vi "FPGA Target_PCIe_7856R.vi"() -> ()   [LabVIEW 2023]
uses:
  <vilib>/Platform/TimedLoop/XDataNode/timing_clust.ctl
  <vilib>/Platform/TimedLoop/XDataNode/nitl_modes.ctl
  <vilib>/Platform/TimedLoop/XDataNode/wakeup.ctl
  <vilib>/rvi/Emulation/niFpgaSctlEmulationGetInTimedLoop.vi
  <vilib>/rvi/Emulation/niFpgaProcessEmulError.vi
  <vilib>/rvi/eio/common/nirviEmuTemplateMethod_errors.vi
  <vilib>/rvi/Emulation/niFpgaGetClockAttributes.vi
  <vilib>/rvi/Emulation/niFpgaEmulationReportErrorSimple.vi
  <vilib>/eio/utilities/niEioResolveVilibRelativePath.vi
  <vilib>/rvi/interface/RandomDataEmulation/niFpgaRandomDataHandleErrors.vi
  <vilib>/rvi/Emulation/niFpgaCriticalErrorInLSC.vi
  Tick Count.vi
  <vilib>/rvi/Memory/Memory_Emulation/nirvimemoryFastEmulation.vi
  <vilib>/rvi/Memory/Memory_Emulation/nirvimemoryEmulation.vi
  <vilib>/rvi/Emulation/niFpgaEmulationIsFPGAContextNoSignature.vi
  <vilib>/rvi/DataTransferAndStorage/Container/Common/niFpgaContainerGetUniqueNameForEmu.vi
  <vilib>/rvi/errors/nirviReportUnexpectedCaseInternalError (U32).vi
  <vilib>/eio/EIONode/EIONode.xnode
  <vilib>/rvi/DataTransferAndStorage/Container/XNode/niFpgaContainer.xnode
  <vilib>/rvi/interface/RandomDataEmulation/nirviRandomDataFpgaReadWriteTemplate.vi
  <vilib>/Platform/TimedLoop/XDataNode/XDataNode.xnode
  <vilib>/rvi/Arithmetic/AddSubMult/XNode/nirviSatArithmetic.xnode
  <vilib>/Platform/TimedLoop/XDataNode/XDNodeRunTimeDep.lvlib
panel:
  out "Move Z Picomotor Direction":bool
  out "Move Z Picomotor":bool
  out "Tick Count(Ticks)":u32
  in  "HoldTimerScale":u64=18446744073709526080
  in  "Feedback1 on  Hold":bool
  out "Feedback2 Error":i32
  out "Feedback1 Error":i32
  out "Feedback2 Boolean":bool
  out "Feedback1 Boolean":bool
  out "ExtraTime 4":fxp<+,64,64>
  in  "DistanceToBulk 3":i16
  in  "DistanceToBulk 2":i16
  out "HasHeldHoldTimeHappend?":bool
  out "Z_axis_-10Vto10V":bool
  out "TraceRetraceFirstUse":bool
  in  "DistanceToBulk":i16
  out "V START":i16
  out "V END":i16
  out "X START":i16
  out "Y START":i16
  out "Z START":i16
  out "X END":i16
  out "Y END":i16
  out "Z END":i16
  out "V2 START":i16
  out "Count Average":i16
  out "AverageSum":i64
  out "IterateHolder":i16
  out "V2 VEl":i16
  out "V2 END":i16
  out "Update Position Loop Wait Time (ms)":u16=1
  out "LineType":i16
  out "V VEl":i16
  out "Z VEL":i16
  out "Y VEL":i16
  out "X VEL":i16
  out "Element":i16
  in  "V on Fly":i16=-32768
  in  "Change V on Fly":bool
  in  "Feedback_Threshold":i64
  in  "FeedBackType":u8
  out "x < y?":bool
  out "ExtraTime 3":fxp<+,64,64>
  in  "P2AvgMinus":i32
  out "ExtraTime 2":fxp<+,64,64>
  in  "P2AvgWhole":i32
  in  "Xoffset":u32
  in  "P":fxp<+/-,32,1>
  in  "Upper limit Of dZ":i32
  in  "FeedBackType 2":u8
  in  "Feedback_Threshold 2":i32
  in  "GreaterThan 2":bool
  in  "GreaterThan":bool
  in  "V2 on Fly":i16=-32768
  in  "Change V on Fly 2":bool
  out "CurrentMeasuredX":i16
  in  "2^(-n)":i16
  out "SampleNum":i16
  in  "Buffer Loop Wait Time (tICKS)":u32=1
  out "SampleIterator":i16
  out "Internal Stop":bool caption="Stop"
  out "MeasuredCurrent":i16=32767
  out "Applied Voltage":i16=-32768
  in  "External Stop":bool caption="Stop"
  in  "External Pause":bool
  out "Applied Z":i16
  out "Applied Y":i16
  out "Applied X":i16
  in  "Internal Pause":bool
  out "Accum Z":i32
  out "Accum I":i32
  out "Accum dV":i32
  out "Accum I2":i32
  out "OnlyStopLineONCE X":bool
  out "Accum Ext ac":i32
  out "Ext amp":i16=32767
  out "Accum Ext phase":i32
  in  "ExpandVelScaller X":i16=-27
  out "LineNumber":u64
  out "WaitingForWayPoints":bool caption="Stop"
  out "HoldTimer (ticks)":u64
  out "MeasuredCurrent 2":i16=32767
  out "Ext Phase":i16=32767
  in  "ExpandVelScaller Y":i16=-27
  in  "ExpandVelScaller Z":i16=-27
  in  "ExpandVelScaller V":i16=-27
  out "Accum I3":i32
  out "MeasuredCurrent 3":i16=32767
  out "MeasuredCurrent 4":i16=32767
  out "Accum Y":i32
  out "Accum X":i32
  out "OnlyStopLineONCE Y":bool
  out "OnlyStopLineONCE Z":bool
  out "OnlyStopLineONCE V":bool
  in  "EndCurrentLine":bool
  out "StopMoveX":bool
  out "StopMoveY":bool
  out "StopMoveZ":bool
  out "StopMoveV":bool
  out "Jump V":bool
  out "Stop Hold Position":bool
  out "Applied Voltage 2":i16
  out "StopMoveV2":bool
  out "Accum dV2":i32
  out "Jump V2":bool
  in  "ExpandVelScaller V2":i16=-27
  out "OnlyStopLineONCE V2":bool
  out "MoveAverage":i16
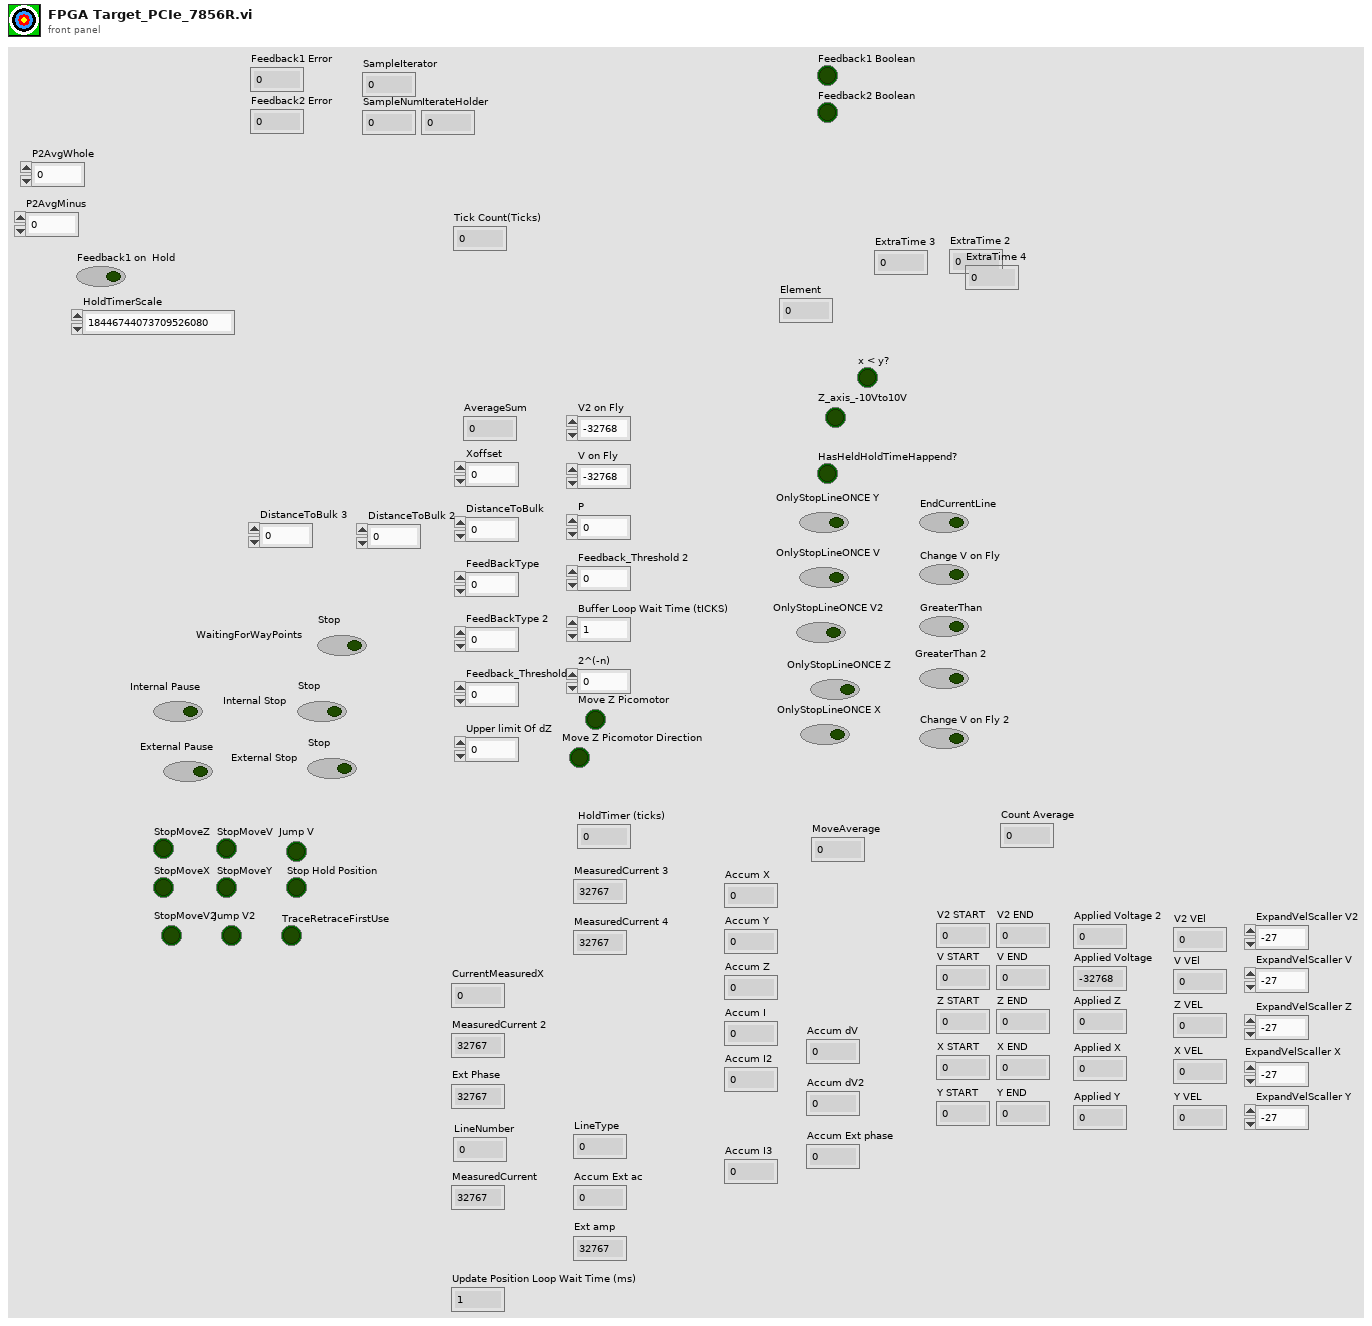
[diagram p1: front panel]
types:
  T1 = typedef "XDNodeRunTimeDep.lvlib/timing_clust.ctl" = cluster{"Expected End [f-1]":u64, "Actual End [f-1]":u64, "Finished Late? [f-1]":bool, "Expected End [i-1]":u64, "Actual End [i-1]":u64, "Finished Late? [i-1]":bool, "Expected Start [i]":u64, "Actual Start [i]":u64, "Expected Start [f]":u64, "Actual Start [f]":u64, "Source Name":string, "Structure Name":string, "Period":i64, "Deadline":i64, "Offset":i64, "Start":i64, "Priority":i32, "Timeout":i32, "Mode":T2, "Wakeup Reason":T3, "Error":errorcluster, "Source Type":string, "Secondary Source Type":string, "Global End Time":u64, "Global Start Time":u64, "Frame Duration":u64, "Iteration Duration":u64, "Assigned CPU":i32, "I/O Scan Engine Mode":u32}
  T2 = typedef "XDNodeRunTimeDep.lvlib/nitl_modes.ctl" = enum32{"No Change", "Process missed periods, maintain original phase", "Discard missed periods, maintain original phase", "Process missed periods, ignore original phase", "Discard missed periods, ignore original phase"}
  T3 = typedef "XDNodeRunTimeDep.lvlib/wakeup.ctl" = enum32{"Normal", "Aborted", "Asynchronous wakeup", "Timing source error", "Timed loop error", "Timeout"}
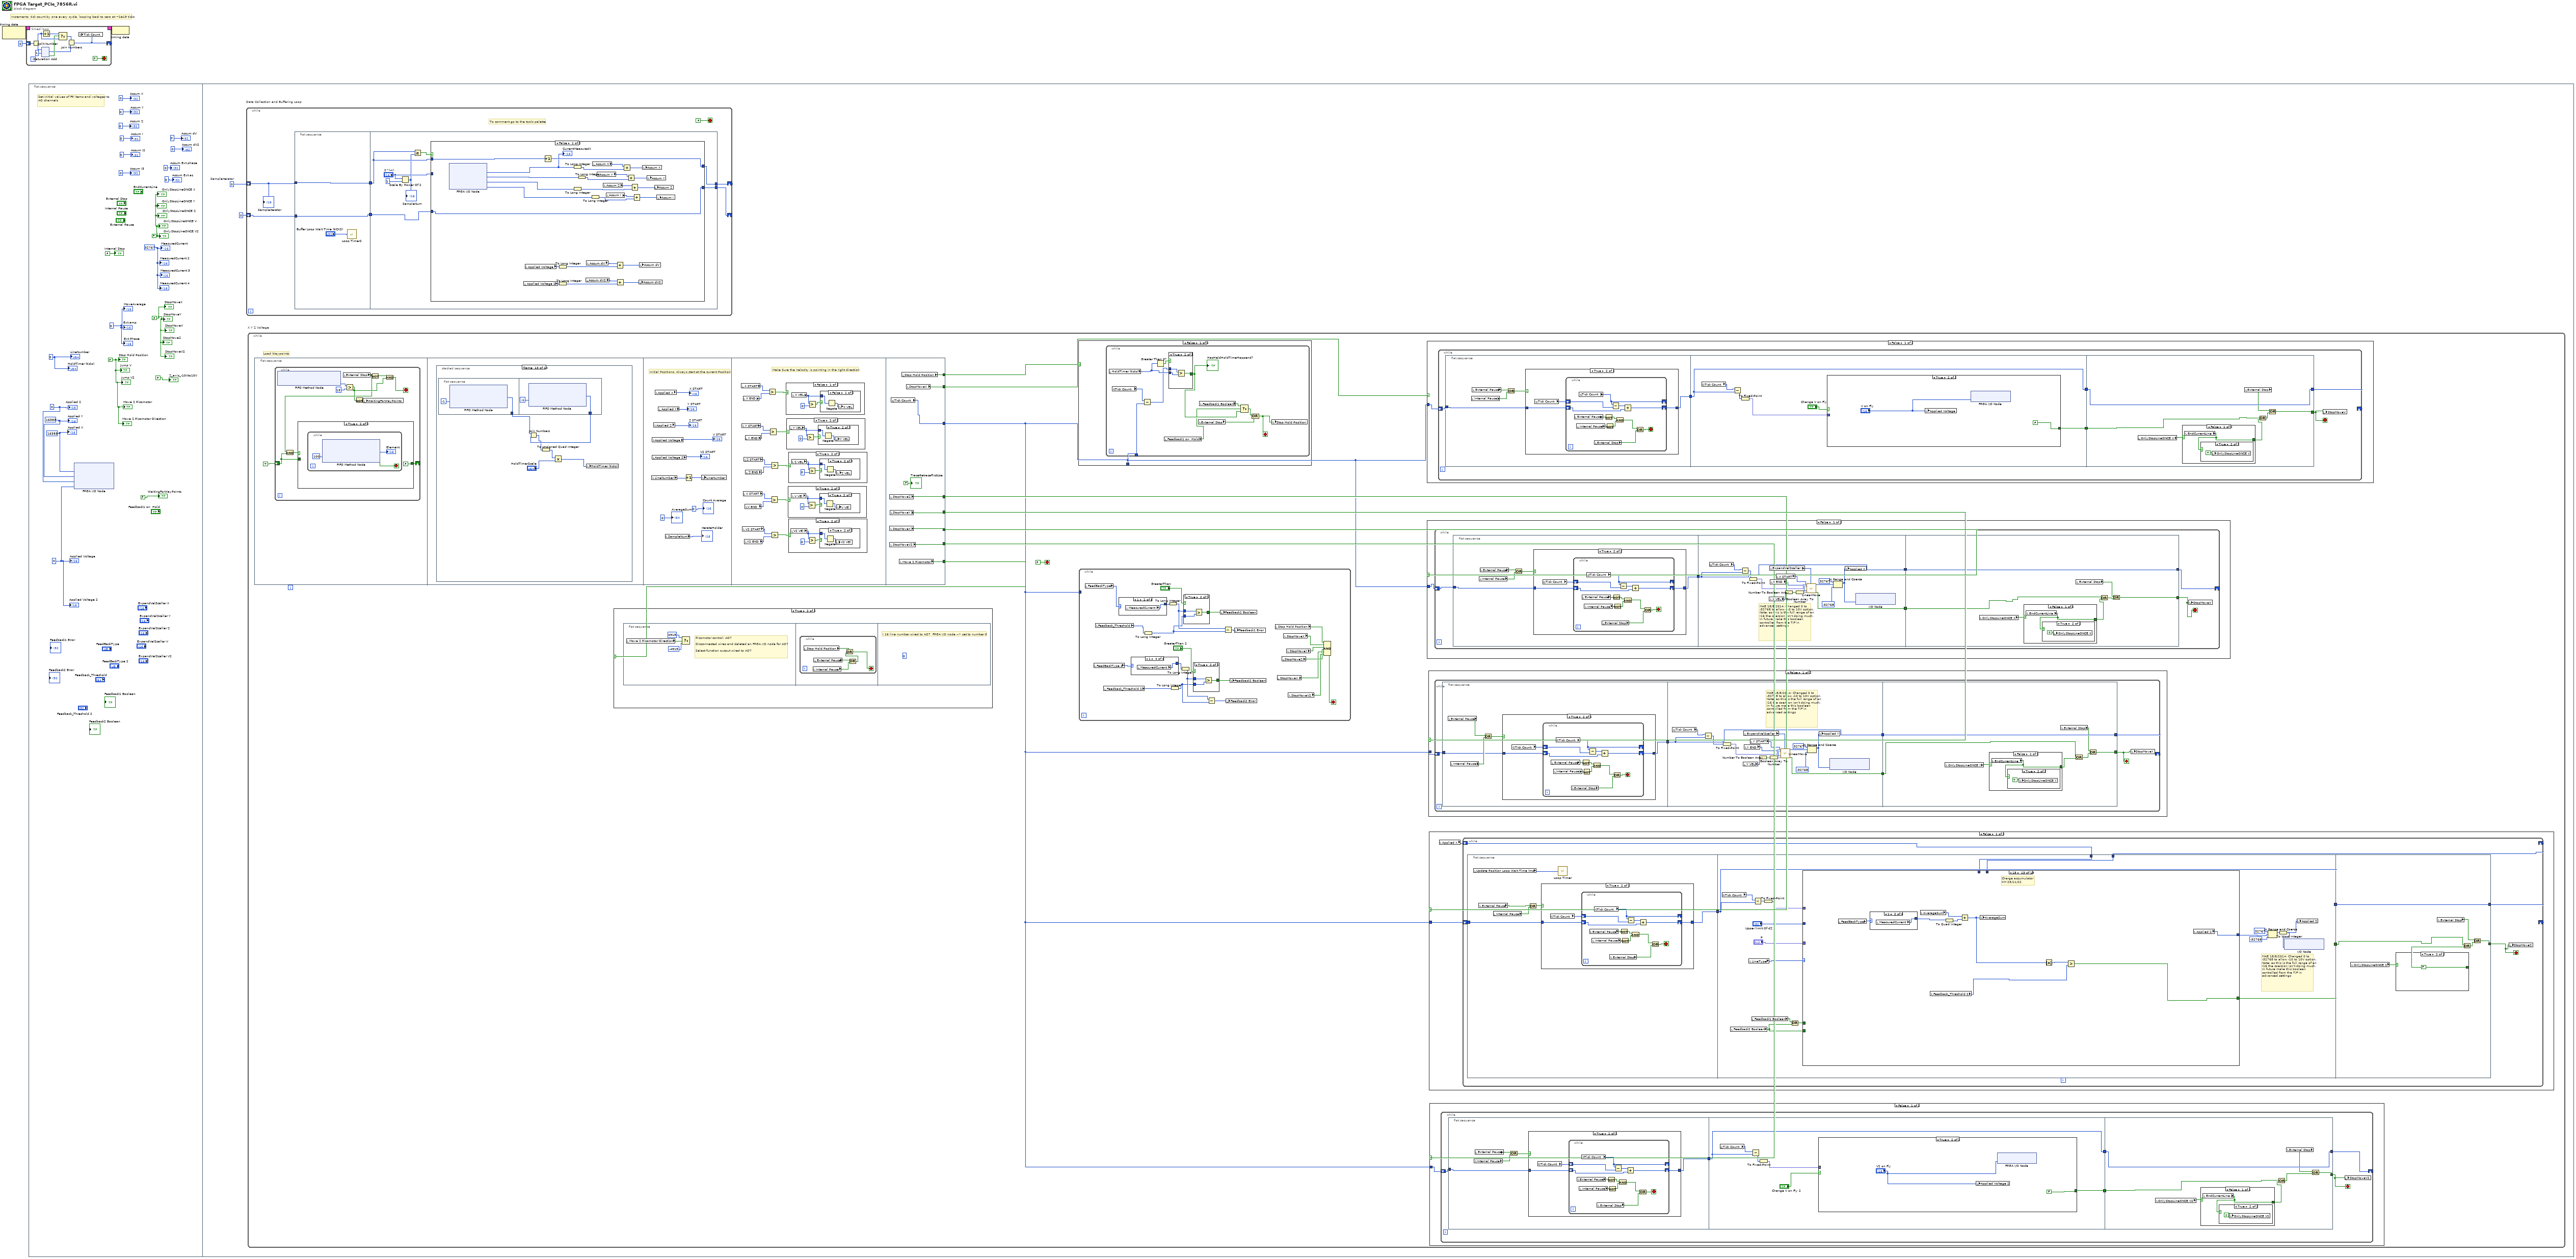
[diagram p0: block diagram]
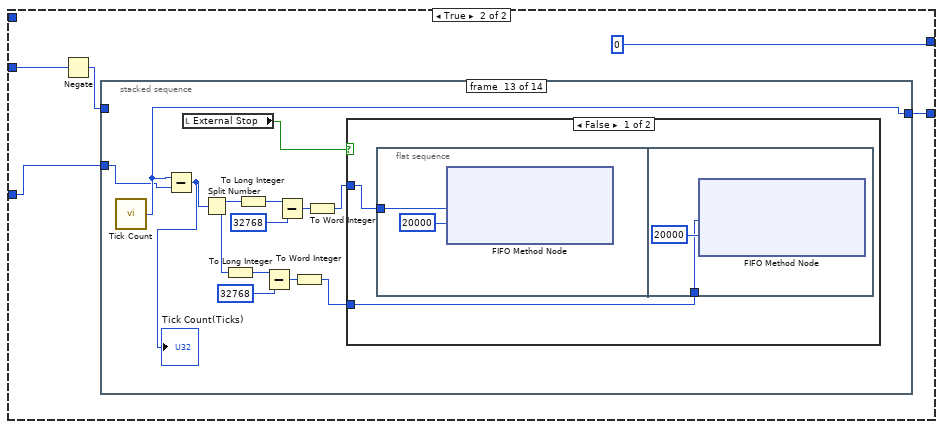
[diagram p2: hidden frame]
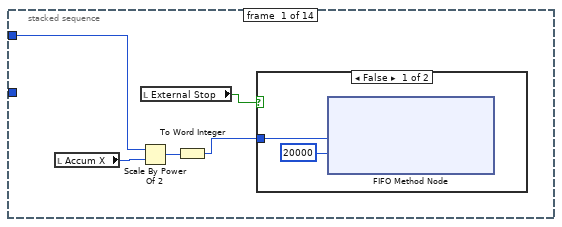
[diagram p3: hidden frame]
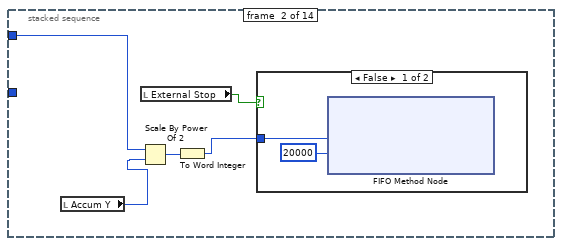
[diagram p5: hidden frame]
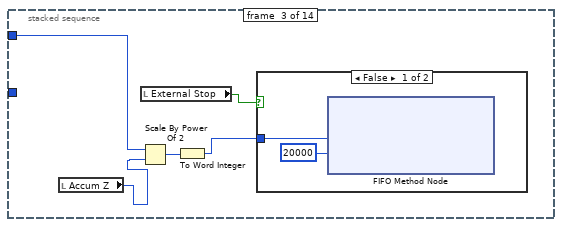
[diagram p7: hidden frame]
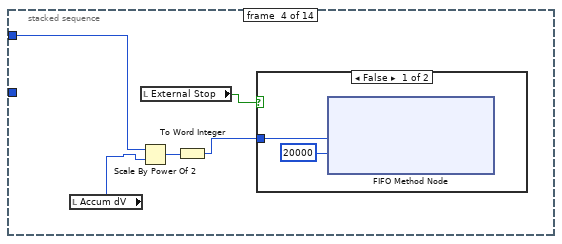
[diagram p9: hidden frame]
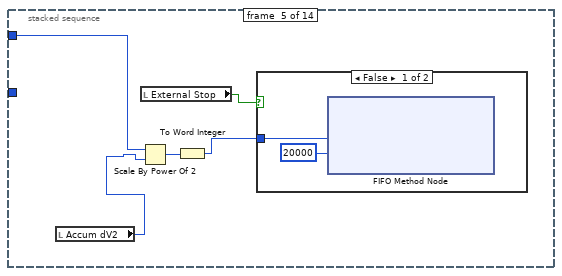
[diagram p11: hidden frame]
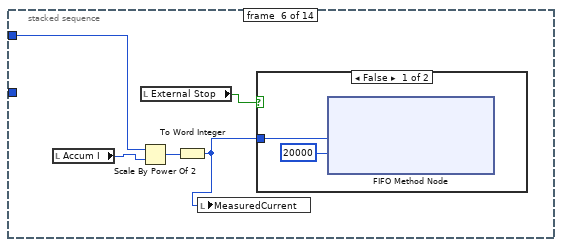
[diagram p13: hidden frame]
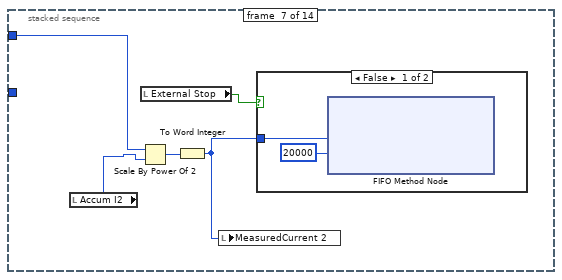
[diagram p15: hidden frame]
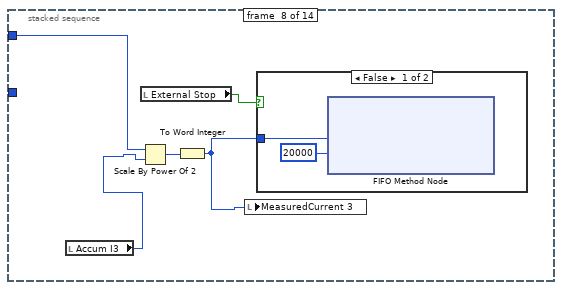
[diagram p17: hidden frame]
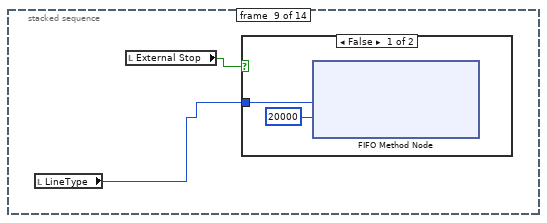
[diagram p19: hidden frame]
diagram:
  # "Increments  tick count by one every cycle, looping back to zero at ~2e19 ticks"
  n1 = node-c288() -> (w3:T1)  [unwired: 1 in]
  n2 = timed-loop {
    timing: w3 -> [_]
    timing-out: [_] -> w2
    shift-right: [w5] -> _
    shift-left: u64 0 -> [w13]
    stop <- FALSE stop-if-true
    n3 = Split Number(x=w13) -> (hi(x)=w10:u32, lo(x)=w12:u32)
    n4 = xnode "Saturation Add"("x"=w12, "y"=u32 1) -> ("x+y"=w6:u32, "overflow"=w7:bool)
    n5 = Increment(x=w10) -> (x+1=w11:u32)
    n6 = Select(t=w11, s=w7, f=w10) -> (s? t:f=w9:u32)
    n7 = Join Numbers(hi=w9, lo=w6) -> ((hi.lo)=w5:u64)
    n8 = global write "Tick Count.vi" "Tick Count"(w5) -> ()
  }
  n9 = flat-sequence {
    frame #0 {
      w33 = FALSE ("OnlyStopLineONCE V2")
      w34 = FALSE ("Internal Stop")
      w29 = FALSE ("Internal Stop")
      w36 = i16 0 ("Applied Volatge")
      w37 = i16 16383 ("Applied Volatge")
      w38 = i16 16383 ("Applied Volatge")
      w32 = u64 0 ("LineNumber")
      w31 = i16 0 ("Ext amp")
      w28 = i16 0 ("Applied Volatge")
      w41 = i16 32767 ("dZ Position")
      # "Set initial values of FP items and voltages to AO channels"
      n10 = xnode "FPGA I/O Node"("Connector0/AO0"=w38, "Connector0/AO1"=w37, "Connector0/AO2"=w36, "Connector0/AO4"=w28) -> ()  [unwired: 4 in, 4 out]
      "Internal Stop" <- FALSE ("Internal Stop")
      "MeasuredCurrent" <- w41
      "Applied Voltage" <- w28
      "Applied Z" <- w36
      "Applied Y" <- w37
      "Applied X" <- w38
      "Accum Z" <- 0 ("Applied Volatge")
      "Accum I" <- 0 ("Applied Volatge")
      "Accum dV" <- 0 ("Applied Volatge")
      "Accum I2" <- 0 ("Applied Volatge")
      "OnlyStopLineONCE X" <- w33
      "Accum Ext ac" <- 0 ("Accum Ext ac")
      "Ext amp" <- w31
      "Accum Ext phase" <- 0 ("Accum Ext phase")
      "LineNumber" <- w32
      "WaitingForWayPoints" <- FALSE ("WaitingForWayPoints")
      "HoldTimer (ticks)" <- w32
      "MeasuredCurrent 2" <- w41
      "Ext Phase" <- w31
      "Accum I3" <- 0 ("Applied Volatge")
      "MeasuredCurrent 3" <- w41
      "MeasuredCurrent 4" <- w41
      "Accum Y" <- 0 ("Applied Volatge")
      "Accum X" <- 0 ("Applied Volatge")
      "OnlyStopLineONCE Y" <- w33
      "OnlyStopLineONCE Z" <- w33
      "OnlyStopLineONCE V" <- w33
      "StopMoveX" <- w34
      "StopMoveY" <- w34
      "StopMoveZ" <- w34
      "StopMoveV" <- w34
      "Jump V" <- w29
      "Stop Hold Position" <- w29
      "Applied Voltage 2" <- w28
      "StopMoveV2" <- w34
      "Accum dV2" <- 0 ("Applied Volatge")
      "Jump V2" <- w29
      "OnlyStopLineONCE V2" <- w33
      "MoveAverage" <- w31
      "Z_axis_-10Vto10V" <- FALSE ("Internal Stop")
      "Move Z Picomotor" <- w29
      "Move Z Picomotor Direction" <- w29
    }
    frame #1 {
      w52 = i16 0  # SampleIterator
      n11 = while "Data Collection and Buffering Loop" {
        shift-right: [w57] -> _
        shift-left: w52 -> [w58]
        shift-right: [w55] -> _
        shift-left: u32 0 ("Tick Count(Ticks)") -> [w53]
        stop <- FALSE stop-if-true
        # "To comment go to the tools palette"
        n12 = flat-sequence {
          tunnel: [w62] -> w59
          tunnel: w58 -> [w62]
          tunnel: w53 -> [w60]
          tunnel: [w60] -> w54
          tunnel: w59 -> [w70]
          tunnel: [w69] -> w57
          tunnel: [w64] -> w55
          tunnel: w54 -> [w63]
          frame #0 {
            n13 = call "Loop Timer2"("Count(Ticks)"="Buffer Loop Wait Time (tICKS)") -> ()  [unwired: 1 out]
          }
          frame #1 {
            n14 = Scale By Power Of 2(n="2^(-n)", x=i16 1) -> (x*2^n=w67:i16)
            "SampleNum" <- w67
            n15 = Greater Or Equal?(x=w70, y=w67) -> (x >= y?=w65:bool)
            n16 = case shown="False" w65 {
              tunnel: w70 -> [w97 _]
              tunnel: [w96 i16 0 ("lo")] -> w69
              tunnel: "2^(-n)" -> [_ w101]
              tunnel: [w72 w99] -> w64
              tunnel: w63 -> [w72 w98]
              frame False {
                n17 = xnode "FPGA I/O Node"() -> ("Connector0/AI0"=w77:i16, "Connector0/AI1"=w84:i16, "Connector0/AI2"=w87:i16, "Connector0/AI4"=w71:i16)  [unwired: 4 in, 4 out]
                "CurrentMeasuredX" <- w77
                n18 = local read "Applied Voltage 2"() -> (w75:i16)
                n19 = local read "Applied Voltage"() -> (w89:i16)
                n20 = Increment(x=w97) -> (x+1=w96:i16)
                n21 = To Long Integer(number=w89) -> (32bit integer=w88:i32)
                n22 = To Long Integer(number=w75) -> (32bit integer=w76:i32)
                n23 = To Long Integer(number=w87) -> (32bit integer=w85:i32)
                n24 = To Long Integer(number=w77) -> (32bit integer=w78:i32)
                n25 = To Long Integer(number=w84) -> (32bit integer=w83:i32)
                n26 = local read "Accum dV2"() -> (w73:i32)
                n27 = local read "Accum dV"() -> (w91:i32)
                n28 = To Long Integer(number=w71) -> (32bit integer=w93:i32)
                n29 = local read "Accum X"() -> (w79:i32)
                n30 = local read "Accum Y"() -> (w82:i32)
                n31 = local read "Accum Z"() -> (w86:i32)
                n32 = local read "Accum I"() -> (w94:i32)
                n33 = Add(x=w91, y=w88) -> (x+y=w90:i32)
                n34 = Add(x=w73, y=w76) -> (x+y=w74:i32)
                n35 = Add(x=w79, y=w78) -> (x+y=w80:i32)
                n36 = Add(x=w82, y=w83) -> (x+y=w81:i32)
                n37 = Add(x=w86, y=w85) -> (x+y=w95:i32)
                n38 = Add(x=w94, y=w93) -> (x+y=w92:i32)
                n39 = local write "Accum dV2"(w74) -> ()
                n40 = local write "Accum dV"(w90) -> ()
                n41 = local write "Accum X"(w80) -> ()
                n42 = local write "Accum Y"(w81) -> ()
                n43 = local write "Accum Z"(w95) -> ()
                n44 = local write "Accum I"(w92) -> ()
              }
              frame True {
                n45 = Negate(x=w101) -> (-x=w100:i16)
                n46 = stacked-sequence {
                  tunnel: w100 -> [w103 w111 w118 w126 w133 w140 w147 w154 _ _ w171 w178 _ _]
                  tunnel: [_ _ _ _ _ _ _ _ _ _ _ _ w184 _] -> w99
                  tunnel: w98 -> [_ _ _ _ _ _ _ _ _ _ _ _ w183 _]
                  frame #0 {
                    n47 = local read "Accum X"() -> (w104:i32)
                    n48 = Scale By Power Of 2(n=w103, x=w104) -> (x*2^n=w105:i32)
                    n49 = local read "External Stop"() -> (w106:bool)
                    n50 = To Word Integer(number=w105) -> (16bit integer=w107:i16)
                    n51 = case shown="False" w106 {
                      tunnel: w107 -> [w108 _]
                      frame False {
                        n52 = xnode ("FIFO Method Node")("Element"=w108, "Timeout"=20000) -> ()  [unwired: 1 in, 2 out]
                      }
                      frame True {
                      }
                    }
                  }
                  frame #1 {
                    n53 = local read "Accum Y"() -> (w110:i32)
                    n54 = Scale By Power Of 2(n=w111, x=w110) -> (x*2^n=w112:i32)
                    n55 = local read "External Stop"() -> (w113:bool)
                    n56 = To Word Integer(number=w112) -> (16bit integer=w114:i16)
                    n57 = case shown="False" w113 {
                      tunnel: w114 -> [w115 _]
                      frame False {
                        n58 = xnode ("FIFO Method Node")("Element"=w115, "Timeout"=20000) -> ()  [unwired: 1 in, 2 out]
                      }
                      frame True {
                      }
                    }
                  }
                  frame #2 {
                    n59 = local read "Accum Z"() -> (w117:i32)
                    n60 = Scale By Power Of 2(n=w118, x=w117) -> (x*2^n=w119:i32)
                    n61 = local read "External Stop"() -> (w120:bool)
                    n62 = To Word Integer(number=w119) -> (16bit integer=w121:i16)
                    n63 = case shown="False" w120 {
                      tunnel: w121 -> [w122 _]
                      frame False {
                        n64 = xnode ("FIFO Method Node")("Element"=w122, "Timeout"=20000) -> ()  [unwired: 1 in, 2 out]
                      }
                      frame True {
                      }
                    }
                  }
                  frame #3 {
                    n65 = local read "Accum dV"() -> (w124:i32)
                    n66 = Scale By Power Of 2(n=w126, x=w124) -> (x*2^n=w127:i32)
                    n67 = local read "External Stop"() -> (w128:bool)
                    n68 = To Word Integer(number=w127) -> (16bit integer=w125:i16)
                    n69 = case shown="False" w128 {
                      tunnel: w125 -> [w129 _]
                      frame False {
                        n70 = xnode ("FIFO Method Node")("Element"=w129, "Timeout"=20000) -> ()  [unwired: 1 in, 2 out]
                      }
                      frame True {
                      }
                    }
                  }
                  frame #4 {
                    n71 = local read "Accum dV2"() -> (w131:i32)
                    n72 = Scale By Power Of 2(n=w133, x=w131) -> (x*2^n=w134:i32)
                    n73 = local read "External Stop"() -> (w135:bool)
                    n74 = To Word Integer(number=w134) -> (16bit integer=w132:i16)
                    n75 = case shown="False" w135 {
                      tunnel: w132 -> [w136 _]
                      frame False {
                        n76 = xnode ("FIFO Method Node")("Element"=w136, "Timeout"=20000) -> ()  [unwired: 1 in, 2 out]
                      }
                      frame True {
                      }
                    }
                  }
                  frame #5 {
                    n77 = local read "Accum I"() -> (w139:i32)
                    n78 = Scale By Power Of 2(n=w140, x=w139) -> (x*2^n=w141:i32)
                    n79 = local read "External Stop"() -> (w142:bool)
                    n80 = To Word Integer(number=w141) -> (16bit integer=w138:i16)
                    n81 = local write "MeasuredCurrent"(w138) -> ()
                    n82 = case shown="False" w142 {
                      tunnel: w138 -> [w143 _]
                      frame False {
                        n83 = xnode ("FIFO Method Node")("Element"=w143, "Timeout"=20000) -> ()  [unwired: 1 in, 2 out]
                      }
                      frame True {
                      }
                    }
                  }
                  frame #6 {
                    n84 = local read "Accum I2"() -> (w146:i32)
                    n85 = Scale By Power Of 2(n=w147, x=w146) -> (x*2^n=w148:i32)
                    n86 = local read "External Stop"() -> (w149:bool)
                    n87 = To Word Integer(number=w148) -> (16bit integer=w145:i16)
                    n88 = local write "MeasuredCurrent 2"(w145) -> ()
                    n89 = case shown="False" w149 {
                      tunnel: w145 -> [w150 _]
                      frame False {
                        n90 = xnode ("FIFO Method Node")("Element"=w150, "Timeout"=20000) -> ()  [unwired: 1 in, 2 out]
                      }
                      frame True {
                      }
                    }
                  }
                  frame #7 {
                    n91 = local read "Accum I3"() -> (w153:i32)
                    n92 = Scale By Power Of 2(n=w154, x=w153) -> (x*2^n=w155:i32)
                    n93 = local read "External Stop"() -> (w156:bool)
                    n94 = To Word Integer(number=w155) -> (16bit integer=w152:i16)
                    n95 = local write "MeasuredCurrent 3"(w152) -> ()
                    n96 = case shown="False" w156 {
                      tunnel: w152 -> [w157 _]
                      frame False {
                        n97 = xnode ("FIFO Method Node")("Element"=w157, "Timeout"=20000) -> ()  [unwired: 1 in, 2 out]
                      }
                      frame True {
                      }
                    }
                  }
                  frame #8 {
                    n98 = local read "LineType"() -> (w159:i16)
                    n99 = local read "External Stop"() -> (w160:bool)
                    n100 = case shown="False" w160 {
                      tunnel: w159 -> [w161 _]
                      frame False {
                        n101 = xnode ("FIFO Method Node")("Element"=w161, "Timeout"=20000) -> ()  [unwired: 1 in, 2 out]
                      }
                      frame True {
                      }
                    }
                  }
                  frame #9 {
                    n102 = local read "LineNumber"() -> (w164:u64)
                    n103 = local read "External Stop"() -> (w165:bool)
                    n104 = To Word Integer(number=w164) -> (16bit integer=w163:i16)
                    n105 = case shown="False" w165 {
                      tunnel: w163 -> [w166 _]
                      frame False {
                        n106 = xnode ("FIFO Method Node")("Element"=w166, "Timeout"=20000) -> ()  [unwired: 1 in, 2 out]
                      }
                      frame True {
                      }
                    }
                  }
                  frame #10 {
                    n107 = local read "Accum Ext ac"() -> (w170:i32)
                    n108 = local read "External Stop"() -> (w172:bool)
                    n109 = Scale By Power Of 2(n=w171, x=w170) -> (x*2^n=w169:i32)
                    n110 = To Word Integer(number=w169) -> (16bit integer=w168:i16)
                    n111 = case shown="False" w172 {
                      tunnel: w168 -> [w173 _]
                      frame False {
                        n112 = xnode ("FIFO Method Node")("Element"=w173, "Timeout"=20000) -> ()  [unwired: 1 in, 2 out]
                      }
                      frame True {
                      }
                    }
                    n113 = local write "Ext amp"(w168) -> ()
                  }
                  frame #11 {
                    n114 = local read "Accum Ext phase"() -> (w176:i32)
                    n115 = local read "External Stop"() -> (w179:bool)
                    n116 = Scale By Power Of 2(n=w178, x=w176) -> (x*2^n=w177:i32)
                    n117 = To Word Integer(number=w177) -> (16bit integer=w175:i16)
                    n118 = local write "Ext Phase"(w175) -> ()
                    n119 = case shown="False" w179 {
                      tunnel: w175 -> [w180 _]
                      frame False {
                        n120 = xnode ("FIFO Method Node")("Element"=w180, "Timeout"=20000) -> ()  [unwired: 1 in, 2 out]
                      }
                      frame True {
                      }
                    }
                  }
                  frame #12 {
                    n121 = call "Tick Count"() -> ("Tick Count(Ticks)"=w184:u32)
                    n122 = Subtract(x=w184, y=w183) -> (x-y=w182:u32)
                    "Tick Count(Ticks)" <- w182
                    n123 = local read "External Stop"() -> (w195:bool)
                    n124 = Split Number(x=w182) -> (hi(x)=w194:u16, lo(x)=w186:u16)
                    n125 = To Long Integer(number=w186) -> (32bit integer=w187:i32)
                    n126 = To Long Integer(number=w194) -> (32bit integer=w193:i32)
                    n127 = Subtract(x=w187, y=32768) -> (x-y=w189:i32)
                    n128 = Subtract(x=w193, y=32768) -> (x-y=w191:i32)
                    n129 = To Word Integer(number=w189) -> (16bit integer=w185:i16)
                    n130 = To Word Integer(number=w191) -> (16bit integer=w190:i16)
                    n131 = case shown="False" w195 {
                      tunnel: w190 -> [w197 _]
                      tunnel: w185 -> [w196 _]
                      frame False {
                        n132 = flat-sequence {
                          tunnel: w197 -> [w198]
                          tunnel: w196 -> [w200]
                          frame #0 {
                            n133 = xnode ("FIFO Method Node")("Element"=w198, "Timeout"=20000) -> ()  [unwired: 1 in, 2 out]
                          }
                          frame #1 {
                            n134 = xnode ("FIFO Method Node")("Element"=w200, "Timeout"=20000) -> ()  [unwired: 1 in, 2 out]
                          }
                        }
                      }
                      frame True {
                      }
                    }
                  }
                  frame #13 {
                    n135 = local write "Accum dV"(0 ("MeasuredCurrent")) -> ()
                    n136 = local write "Accum Z"(0 ("MeasuredCurrent")) -> ()
                    n137 = local write "Accum dV2"(0 ("Accum Ext ac")) -> ()
                    n138 = local write "Accum I2"(0 ("MeasuredCurrent")) -> ()
                    n139 = local write "Accum I"(0 ("MeasuredCurrent")) -> ()
                    n140 = local write "Accum Y"(0 ("Accum Ext ac")) -> ()
                    n141 = local write "Accum X"(0 ("MeasuredCurrent")) -> ()
                    n142 = local write "Accum Ext ac"(0 ("Accum Ext ac")) -> ()
                    n143 = local write "Accum I3"(0 ("Accum Ext ac")) -> ()
                    n144 = local write "Accum Ext phase"(0 ("Accum Ext phase")) -> ()
                  }
                }
              }
            }
          }
        }
        "SampleIterator" <- w58
      }
      n145 = while "X Y Z Voltage" {
        stop <- FALSE stop-if-true
        # "Load Waypoints"
        n146 = flat-sequence {
          tunnel: [w1138] -> w213
          tunnel: [w1137] -> w219
          tunnel: [w1136] -> w218
          tunnel: [w1135] -> w217
          tunnel: [w1134] -> w216
          tunnel: [w1133] -> w215
          tunnel: [w1131] -> w214
          tunnel: [w1130] -> w212
          frame #0 {
            n147 = while {
              shift-right: [w934] -> _
              shift-left: TRUE ("WaitingForWayPoints") -> [w935]
              stop <- w938 stop-if-true
              n148 = xnode ("FIFO Method Node")() -> ("Number of Elements to Read"=w943:u32)  [unwired: 1 in, 1 out]
              n149 = local read "External Stop"() -> (w936:bool)
              n150 = And(x=w936, y=w935) -> (x .and. y?=w937:bool)
              n151 = case shown="True" w937 {
                tunnel: w935 -> [w944 _]
                tunnel: [w944 FALSE ("WaitingForWayPoints")] -> w934
                frame False {
                }
                frame True {
                  n152 = while {
                    stop <- w946 stop-if-true
                    n153 = xnode ("FIFO Method Node")("Timeout"=100) -> ("Element"=→"Element":i16, "Timed Out?"=w946:bool)  [unwired: 1 in, 1 out]
                  }
                }
              }
              n154 = Greater?(x=w943, y=u32 13) -> (0:w939:bool)
              n155 = Not(x=w939) -> (.not. x?=w941:bool)
              n156 = local write "WaitingForWayPoints"(w941) -> ()
              n157 = Not(x=w936) -> (.not. x?=w940:bool)
              n158 = And(x=w940, y=w939) -> (x .and. y?=w938:bool)
            }
          }
          frame #1 {
            n159 = stacked-sequence {
              frame #0 {
                n160 = xnode ("FIFO Method Node")("Timeout"=-1) -> ("Element"=→"LineType":i16)  [unwired: 1 in, 2 out]
              }
              frame #1 {
                n161 = xnode ("FIFO Method Node")("Timeout"=-1) -> ("Element"=→"X VEL":i16)  [unwired: 1 in, 2 out]
              }
              frame #2 {
                n162 = xnode ("FIFO Method Node")("Timeout"=-1) -> ("Element"=→"Y VEL":i16)  [unwired: 1 in, 2 out]
              }
              frame #3 {
                n163 = xnode ("FIFO Method Node")("Timeout"=-1) -> ("Element"=→"Z VEL":i16)  [unwired: 1 in, 2 out]
              }
              frame #4 {
                n164 = xnode ("FIFO Method Node")("Timeout"=-1) -> ("Element"=→"V VEl":i16)  [unwired: 1 in, 2 out]
              }
              frame #5 {
                n165 = xnode ("FIFO Method Node")("Timeout"=-1) -> ("Element"=→"V2 VEl":i16)  [unwired: 1 in, 2 out]
              }
              frame #6 {
                n166 = xnode ("FIFO Method Node")("Timeout"=-1) -> ("Element"=→"X END":i16)  [unwired: 1 in, 2 out]
              }
              frame #7 {
                n167 = xnode ("FIFO Method Node")("Timeout"=-1) -> ("Element"=→"Y END":i16)  [unwired: 1 in, 2 out]
              }
              frame #8 {
                n168 = xnode ("FIFO Method Node")("Timeout"=-1) -> ("Element"=w966:i16)  [unwired: 1 in, 2 out]
                n169 = local read "LineType"() -> (w967:i16)
                n170 = case shown="13" w967 {
                  tunnel: [w969 w974 w986 w998 w1006] -> w965
                  tunnel: w966 -> [w969 _ _ _ _]
                  frame 0..2, Default {
                    # "Normal Move"
                  }
                  frame 3 {
                    # "Bulk At End Of line - Retract"
                    n171 = local read "Z_axis_-10Vto10V"() -> (w973:bool)
                    n172 = local read "Applied Z"() -> (w981:i16)
                    n173 = Select(t=-32768 ("lower limit"), s=w973, f=0 ("lower limit")) -> (s? t:f=w972:i32)
                    n174 = To Long Integer(number=w981) -> (32bit integer=w978:i32)
                    n175 = To Long Integer(number="DistanceToBulk") -> (32bit integer=w979:i32)
                    n176 = Add(x=w978, y=w979) -> (x+y=w977:i32)
                    n177 = In Range and Coerce(upper limit=32767, x=w977, lower limit=w972) -> (coerced(x)=w975:i32)  [unwired: 1 out]
                    n178 = To Word Integer(number=w975) -> (16bit integer=w974:i16)
                  }
                  frame 12 {
                    # "Bulk At End Of line - Retract"
                    n179 = local read "Z_axis_-10Vto10V"() -> (w985:bool)
                    n180 = local read "Applied Z"() -> (w993:i16)
                    n181 = Select(t=-32768 ("lower limit"), s=w985, f=0 ("lower limit")) -> (s? t:f=w984:i32)
                    n182 = To Long Integer(number=w993) -> (32bit integer=w990:i32)
                    n183 = To Long Integer(number="DistanceToBulk 2") -> (32bit integer=w991:i32)
                    n184 = Add(x=w990, y=w991) -> (x+y=w989:i32)
                    n185 = In Range and Coerce(upper limit=32767, x=w989, lower limit=w984) -> (coerced(x)=w987:i32)  [unwired: 1 out]
                    n186 = To Word Integer(number=w987) -> (16bit integer=w986:i16)
                  }
                  frame 13 {
                    # "Bulk At End Of line - Retract"
                    n187 = local read "Z_axis_-10Vto10V"() -> (w997:bool)
                    n188 = local read "Applied Z"() -> (w1005:i16)
                    n189 = Select(t=-32768 ("lower limit"), s=w997, f=0 ("lower limit")) -> (s? t:f=w996:i32)
                    n190 = To Long Integer(number=w1005) -> (32bit integer=w1002:i32)
                    n191 = To Long Integer(number="DistanceToBulk 3") -> (32bit integer=w1003:i32)
                    n192 = Add(x=w1002, y=w1003) -> (x+y=w1001:i32)
                    n193 = In Range and Coerce(upper limit=32767, x=w1001, lower limit=w996) -> (coerced(x)=w999:i32)  [unwired: 1 out]
                    n194 = To Word Integer(number=w999) -> (16bit integer=w998:i16)
                  }
                  frame 4..7 {
                    # "Start at current hieght"
                    n195 = local read "Applied Z"() -> (w1006:i16)
                  }
                }
                "Z END" <- w965
              }
              frame #9 {
                n196 = xnode ("FIFO Method Node")("Timeout"=-1) -> ("Element"=→"V END":i16)  [unwired: 1 in, 2 out]
              }
              frame #10 {
                n197 = xnode ("FIFO Method Node")("Timeout"=-1) -> ("Element"=→"V2 END":i16)  [unwired: 1 in, 2 out]
              }
              frame #11 {
                n198 = xnode ("FIFO Method Node")("Timeout"=-1) -> ("Element"=w1012:i16)  [unwired: 1 in, 2 out]
                n199 = To Unsigned Word Integer(number=w1012) -> (unsigned 16bit integer=→"Update Position Loop Wait Time (ms)":u16)
              }
              frame #12 {
                n200 = flat-sequence {
                  tunnel: [w1020] -> w1016
                  tunnel: [w1022] -> w1015
                  frame #0 {
                    n201 = xnode ("FIFO Method Node")("Timeout"=-1) -> ("Element"=w1020:i16)  [unwired: 1 in, 2 out]
                  }
                  frame #1 {
                    n202 = xnode ("FIFO Method Node")("Timeout"=-1) -> ("Element"=w1022:i16)  [unwired: 1 in, 2 out]
                  }
                }
                n203 = Join Numbers(hi=w1016, lo=w1015) -> ((hi.lo)=w1014:u32)
                n204 = To Unsigned Quad Integer(1:w1014) -> (0:w1019:u64)
                n205 = Multiply(x=w1019, y="HoldTimerScale") -> (x*y=w1017:u64)
                n206 = local write "HoldTimer (ticks)"(w1017) -> ()
              }
              frame #13 {
                n207 = xnode ("FIFO Method Node")("Timeout"=-1) -> ("Element"=w1033:i16)  [unwired: 1 in, 2 out]
                n208 = Number To Boolean Array(number=w1033) -> (Boolean array=w1024:bool[])
                n209 = Index Array(array=w1024, index=0) -> (element=w1038:bool)
                n210 = Index Array(array=w1024, index=1) -> (element=w1039:bool)
                n211 = Index Array(array=w1024, index=2) -> (element=w1043:bool)
                n212 = Index Array(array=w1024, index=4) -> (element=w1048:bool)
                n213 = Index Array(array=w1024, index=5) -> (element=w1032:bool)
                n214 = Index Array(array=w1024, index=3) -> (element=w1040:bool)
                n215 = Index Array(array=w1024, index=10) -> (element=w1026:bool)
                n216 = Index Array(array=w1024, index=9) -> (element=w1027:bool)
                n217 = Index Array(array=w1024, index=6) -> (element=w1050:bool)
                n218 = Not(x=w1040) -> (.not. x?=w1047:bool)
                n219 = Not(x=w1038) -> (.not. x?=w1044:bool)
                n220 = Not(x=w1032) -> (.not. x?=w1031:bool)
                n221 = Index Array(array=w1024, index=7) -> (element=w1053:bool)
                n222 = Index Array(array=w1024, index=8) -> (element=w1029:bool)
                n223 = Not(x=w1043) -> (.not. x?=w1046:bool)
                n224 = Not(x=w1039) -> (.not. x?=w1045:bool)
                n225 = local write "StopMoveX"(w1044) -> ()
                n226 = local write "Stop Hold Position"(w1031) -> ()
                n227 = Not(x=w1050) -> (.not. x?=w1051:bool)
                n228 = local write "Move Z Picomotor Direction"(w1026) -> ()
                n229 = local write "StopMoveY"(w1045) -> ()
                n230 = local write "StopMoveZ"(w1046) -> ()
                n231 = local write "StopMoveV2"(w1051) -> ()
                n232 = local write "StopMoveV"(w1047) -> ()
                n233 = local write "Move Z Picomotor"(w1027) -> ()
                n234 = local write "Jump V"(w1048) -> ()
                n235 = local write "Feedback1 on  Hold"(w1029) -> ()
                n236 = local write "Jump V2"(w1053) -> ()
              }
            }
          }
          frame #2 {
            # "Initial Positions, Always start at the current Position"
            n237 = local read "LineNumber"() -> (w1060:u64)
            n238 = local read "Applied Voltage"() -> (→"V START":i16)
            n239 = local read "Applied Voltage 2"() -> (→"V2 START":i16)
            n240 = local read "Applied Z"() -> (→"Z START":i16)
            n241 = local read "Applied X"() -> (→"X START":i16)
            n242 = local read "Applied Y"() -> (→"Y START":i16)
            n243 = local read "SampleNum"() -> (→"IterateHolder":i16)
            n244 = Increment(x=w1060) -> (x+1=w1059:u64)
            n245 = local write "LineNumber"(w1059) -> ()
            "Count Average" <- i16 0
            "AverageSum" <- i64 0 ("LineNumber")
          }
          frame #3 {
            # "Make Sure the Velocity is pointing in the right direction"
            n246 = local read "X START"() -> (w1079:i16)
            n247 = local read "Y START"() -> (w1074:i16)
            n248 = local read "V2 START"() -> (w1067:i16)
            n249 = local read "X END"() -> (w1078:i16)
            n250 = local read "V START"() -> (w1068:i16)
            n251 = local read "Z START"() -> (w1073:i16)
            n252 = local read "V2 END"() -> (w1066:i16)
            n253 = local read "V END"() -> (w1069:i16)
            n254 = local read "Y END"() -> (w1075:i16)
            n255 = local read "Z END"() -> (w1072:i16)
            n256 = Greater?(x=w1079, y=w1078) -> (0:w1077:bool)
            n257 = Greater?(x=w1074, y=w1075) -> (0:w1076:bool)
            n258 = Greater?(x=w1068, y=w1069) -> (0:w1070:bool)
            n259 = Greater?(x=w1073, y=w1072) -> (0:w1071:bool)
            n260 = Greater?(x=w1067, y=w1066) -> (0:w1065:bool)
            n261 = case shown="False" w1077 {
              frame False {
                n262 = local read "X VEL"() -> (w1120:i16)
                n263 = Greater?(x=w1120, y=i16 0) -> (0:w1121:bool)
                n264 = case shown="False" w1121 {
                  tunnel: w1120 -> [w1124 _]
                  frame False {
                    n265 = Negate(x=w1124) -> (-x=w1123:i16)
                    n266 = local write "X VEL"(w1123) -> ()
                  }
                  frame True {
                  }
                }
              }
              frame True {
                n267 = local read "X VEL"() -> (w1125:i16)
                n268 = Greater?(x=w1125, y=i16 0) -> (0:w1126:bool)
                n269 = case shown="True" w1126 {
                  tunnel: w1125 -> [_ w1129]
                  frame False {
                  }
                  frame True {
                    n270 = Negate(x=w1129) -> (-x=w1128:i16)
                    n271 = local write "X VEL"(w1128) -> ()
                  }
                }
              }
            }
            n272 = case shown="True" w1076 {
              frame False {
                n273 = local read "Y VEL"() -> (w1110:i16)
                n274 = Greater?(x=w1110, y=i16 0) -> (0:w1111:bool)
                n275 = case shown="False" w1111 {
                  tunnel: w1110 -> [w1114 _]
                  frame False {
                    n276 = Negate(x=w1114) -> (-x=w1113:i16)
                    n277 = local write "Y VEL"(w1113) -> ()
                  }
                  frame True {
                  }
                }
              }
              frame True {
                n278 = local read "Y VEL"() -> (w1115:i16)
                n279 = Greater?(x=w1115, y=i16 0) -> (0:w1116:bool)
                n280 = case shown="True" w1116 {
                  tunnel: w1115 -> [_ w1119]
                  frame False {
                  }
                  frame True {
                    n281 = Negate(x=w1119) -> (-x=w1118:i16)
                    n282 = local write "Y VEL"(w1118) -> ()
                  }
                }
              }
            }
            n283 = case shown="True" w1070 {
              frame False {
                n284 = local read "V VEl"() -> (w1090:i16)
                n285 = Greater?(x=w1090, y=i16 0) -> (0:w1091:bool)
                n286 = case shown="False" w1091 {
                  tunnel: w1090 -> [w1094 _]
                  frame False {
                    n287 = Negate(x=w1094) -> (-x=w1093:i16)
                    n288 = local write "V VEl"(w1093) -> ()
                  }
                  frame True {
                  }
                }
              }
              frame True {
                n289 = local read "V VEl"() -> (w1095:i16)
                n290 = Greater?(x=w1095, y=i16 0) -> (0:w1096:bool)
                n291 = case shown="True" w1096 {
                  tunnel: w1095 -> [_ w1099]
                  frame False {
                  }
                  frame True {
                    n292 = Negate(x=w1099) -> (-x=w1098:i16)
                    n293 = local write "V VEl"(w1098) -> ()
                  }
                }
              }
            }
            n294 = case shown="True" w1071 {
              frame False {
                n295 = local read "Z VEL"() -> (w1100:i16)
                n296 = Greater?(x=w1100, y=i16 0) -> (0:w1101:bool)
                n297 = case shown="False" w1101 {
                  tunnel: w1100 -> [w1104 _]
                  frame False {
                    n298 = Negate(x=w1104) -> (-x=w1103:i16)
                    n299 = local write "Z VEL"(w1103) -> ()
                  }
                  frame True {
                  }
                }
              }
              frame True {
                n300 = local read "Z VEL"() -> (w1105:i16)
                n301 = Greater?(x=w1105, y=i16 0) -> (0:w1106:bool)
                n302 = case shown="True" w1106 {
                  tunnel: w1105 -> [_ w1109]
                  frame False {
                  }
                  frame True {
                    n303 = Negate(x=w1109) -> (-x=w1108:i16)
                    n304 = local write "Z VEL"(w1108) -> ()
                  }
                }
              }
            }
            n305 = case shown="True" w1065 {
              frame False {
                n306 = local read "V2 VEl"() -> (w1080:i16)
                n307 = Greater?(x=w1080, y=i16 0) -> (0:w1081:bool)
                n308 = case shown="False" w1081 {
                  tunnel: w1080 -> [w1084 _]
                  frame False {
                    n309 = Negate(x=w1084) -> (-x=w1083:i16)
                    n310 = local write "V2 VEl"(w1083) -> ()
                  }
                  frame True {
                  }
                }
              }
              frame True {
                n311 = local read "V2 VEl"() -> (w1085:i16)
                n312 = Greater?(x=w1085, y=i16 0) -> (0:w1086:bool)
                n313 = case shown="True" w1086 {
                  tunnel: w1085 -> [_ w1089]
                  frame False {
                  }
                  frame True {
                    n314 = Negate(x=w1089) -> (-x=w1088:i16)
                    n315 = local write "V2 VEl"(w1088) -> ()
                  }
                }
              }
            }
          }
          frame #4 {
            n316 = local read "StopMoveZ"() -> (w1134:bool)
            n317 = local read "StopMoveX"() -> (w1136:bool)
            n318 = local read "StopMoveV2"() -> (w1133:bool)
            n319 = local read "StopMoveY"() -> (w1135:bool)
            n320 = global read "Tick Count.vi" "Tick Count"() -> (w1138:u64)
            n321 = local read "Move Z Picomotor"() -> (w1130:bool)
            n322 = local read "Stop Hold Position"() -> (w1131:bool)
            n323 = local read "StopMoveV"() -> (w1137:bool)
            "TraceRetraceFirstUse" <- FALSE ("Boolean")
          }
        }
        n324 = case shown="True" w212 {
          frame False {
          }
          frame True {
            n325 = flat-sequence {
              frame #0 {
                # "Picomotor control: AO7\n\nDisconnected wires and deleted an FPGA I/O node for AO7\n\nSelect function output wired to AO7"
                n326 = local read "Move Z Picomotor Direction"() -> (w221:bool)
                n327 = Select(t=i16 4915 ("LineNumber"), s=w221, f=i16 -4915 ("LineNumber")) -> ()  [unwired: 1 out]
              }
              frame #1 {
                n328 = while {
                  stop <- w224 stop-if-true
                  n329 = local read "Stop Hold Position"() -> (w228:bool)
                  n330 = local read "Internal Pause"() -> (w227:bool)
                  n331 = local read "External Pause"() -> (w226:bool)
                  n332 = Or(x=w226, y=w227) -> (x .or. y?=w225:bool)
                  n333 = Or(x=w228, y=w225) -> (x .or. y?=w224:bool)
                }
              }
              frame #2 {
                (unwired) i16 0 ("LineNumber")
                # "I 16 line number wired to AO7  FPGA I/O node --> set to number 0"
              }
            }
          }
        }
        n334 = case shown="False" w214 {
          tunnel: w213 -> [w276 _]
          frame False {
            n335 = while {
              tunnel: w276 -> [w284]
              stop <- w280 stop-if-true
              n336 = local read "HoldTimer (ticks)"() -> (w286:u64)
              n337 = global read "Tick Count.vi" "Tick Count"() -> (w285:u64)
              n338 = Subtract(x=w285, y=w284) -> (x-y=w283:u64)
              n339 = Greater Than 0?(x=w286) -> (x > 0?=w287:bool)
              n340 = local read "Feedback1 on  Hold"() -> (w277:bool)
              n341 = case shown="True" w287 {
                tunnel: [FALSE w291] -> w278
                tunnel: w286 -> [_ w290]
                tunnel: w283 -> [_ w289]
                frame False {
                }
                frame True {
                  n342 = Greater?(x=w289, y=w290) -> (0:w291:bool)
                }
              }
              "HasHeldHoldTimeHappend?" <- w278
              n343 = local read "External Stop"() -> (w281:bool)
              n344 = local read "Feedback1 Boolean"() -> (w282:bool)
              n345 = Select(t=w282, s=w277, f=w278) -> (s? t:f=w279:bool)
              n346 = Compound Arithmetic op=OR(w279, w281) -> (w280:bool)
              n347 = local write "Stop Hold Position"(w280) -> ()
            }
          }
          frame True {
          }
        }
        n348 = while {
          tunnel: w213 -> [_]
          stop <- w238 stop-if-true
          n349 = local read "FeedBackType"() -> (w250:u8)
          n350 = local read "FeedBackType 2"() -> (w248:u8)
          n351 = local read "Feedback_Threshold"() -> (w232:i64)
          n352 = local read "Feedback_Threshold 2"() -> (w230:i32)
          n353 = case shown="1" w250 {
            tunnel: [w270 w271 w272 w273 w274 w275] -> w251
            frame 0, Default {
              n354 = local read "Ext amp"() -> (w270:i16)
            }
            frame 1 {
              n355 = local read "MeasuredCurrent"() -> (w271:i16)
            }
            frame 2 {
              n356 = local read "MeasuredCurrent 2"() -> (w272:i16)
            }
            frame 3 {
              n357 = local read "Ext Phase"() -> (w273:i16)
            }
            frame 4 {
              n358 = local read "MeasuredCurrent"() -> (w274:i16)
            }
            frame 5 {
              n359 = local read "MeasuredCurrent 2"() -> (w275:i16)
            }
          }
          n360 = case shown="1" w248 {
            tunnel: [w258 w259 w260 w261 w262 w263] -> w246
            frame 0, Default {
              n361 = local read "Ext amp"() -> (w258:i16)
            }
            frame 4 {
              n362 = local read "MeasuredCurrent 3"() -> (w259:i16)
            }
            frame 5 {
              n363 = local read "MeasuredCurrent 4"() -> (w260:i16)
            }
            frame 1 {
              n364 = local read "MeasuredCurrent"() -> (w261:i16)
            }
            frame 2 {
              n365 = local read "MeasuredCurrent 2"() -> (w262:i16)
            }
            frame 3 {
              n366 = local read "Ext Phase"() -> (w263:i16)
            }
          }
          n367 = To Long Integer(number=w232) -> (32bit integer=w231:i32)
          n368 = To Long Integer(number=w251) -> (32bit integer=w236:i32)
          n369 = To Long Integer(number=w230) -> (32bit integer=w229:i32)
          n370 = To Long Integer(number=w246) -> (32bit integer=w234:i32)
          n371 = case shown="True" "GreaterThan" {
            tunnel: w236 -> [w266 w269]
            tunnel: w231 -> [w265 w267]
            tunnel: [w264 w268] -> w245
            frame False {
              n372 = Less?(x=w266, y=w265) -> (x < y?=w264:bool)
            }
            frame True {
              n373 = Greater?(x=w269, y=w267) -> (0:w268:bool)
            }
          }
          n374 = case shown="True" "GreaterThan 2" {
            tunnel: w234 -> [w254 w257]
            tunnel: w229 -> [w253 w255]
            tunnel: [w252 w256] -> w244
            frame False {
              n375 = Less?(x=w254, y=w253) -> (x < y?=w252:bool)
            }
            frame True {
              n376 = Greater?(x=w257, y=w255) -> (0:w256:bool)
            }
          }
          n377 = Subtract(x=w234, y=w229) -> (x-y=w233:i32)
          n378 = local write "Feedback1 Boolean"(w245) -> ()
          n379 = Subtract(x=w236, y=w231) -> (x-y=w235:i32)
          n380 = local write "Feedback2 Error"(w233) -> ()
          n381 = local write "Feedback2 Boolean"(w244) -> ()
          n382 = local write "Feedback1 Error"(w235) -> ()
          n383 = local read "Stop Hold Position"() -> (w237:bool)
          n384 = local read "StopMoveV"() -> (w240:bool)
          n385 = local read "StopMoveZ"() -> (w241:bool)
          n386 = local read "StopMoveX"() -> (w243:bool)
          n387 = local read "StopMoveY"() -> (w242:bool)
          n388 = local read "StopMoveV2"() -> (w239:bool)
          n389 = Compound Arithmetic op=AND(w237, w243, w242, w241, w240, w239) -> (w238:bool)
        }
        n390 = case shown="False" w219 {
          tunnel: w213 -> [w871 _]
          frame False {
            n391 = while {
              shift-right: [w873] -> _
              shift-left: w871 -> [w876]
              stop <- w872 stop-if-true
              n392 = flat-sequence {
                tunnel: w876 -> [w878]
                tunnel: [w879] -> w877
                tunnel: w877 -> [w904]
                tunnel: [w904] -> w875
                tunnel: [w900] -> w874
                tunnel: [w929] -> w873
                tunnel: w875 -> [w929]
                tunnel: w874 -> [w923]
                tunnel: [w924] -> w872
                frame #0 {
                  n393 = local read "Internal Pause"() -> (w881:bool)
                  n394 = local read "External Pause"() -> (w882:bool)
                  n395 = Or(x=w882, y=w881) -> (x .or. y?=w880:bool)
                  n396 = case shown="True" w880 {
                    tunnel: w878 -> [w883 w886]
                    tunnel: [w883 w884] -> w879
                    frame False {
                    }
                    frame True {
                      n397 = global read "Tick Count.vi" "Tick Count"() -> (w885:u64)
                      n398 = while {
                        shift-right: [w898] -> w884
                        shift-left: w886 -> [w890]
                        shift-right: [w893] -> _
                        shift-left: w885 -> [w892]
                        stop <- w887 stop-if-true
                        n399 = local read "External Pause"() -> (w897:bool)
                        n400 = local read "Internal Pause"() -> (w895:bool)
                        n401 = global read "Tick Count.vi" "Tick Count"() -> (w893:u64)
                        n402 = local read "External Stop"() -> (w889:bool)
                        n403 = Not(x=w897) -> (.not. x?=w896:bool)
                        n404 = Not(x=w895) -> (.not. x?=w894:bool)
                        n405 = Subtract(x=w893, y=w892) -> (x-y=w891:u64)
                        n406 = And(x=w896, y=w894) -> (x .and. y?=w888:bool)
                        n407 = Add(x=w891, y=w890) -> (x+y=w898:u64)
                        n408 = Or(x=w888, y=w889) -> (x .or. y?=w887:bool)
                      }
                    }
                  }
                }
                frame #1 {
                  n409 = global read "Tick Count.vi" "Tick Count"() -> (w903:u64)
                  n410 = Subtract(x=w903, y=w904) -> (x-y=w901:u64)
                  n411 = To Fixed-Point(number=w901) -> (fixed-point=w902:fxp<+,64,64>)  [unwired: 1 in]
                  n412 = case shown="True" "Change V on Fly" {
                    tunnel: w902 -> [w909 _]
                    tunnel: [w908 FALSE ("Finished Move")] -> w900
                    frame False {
                      n413 = local read "Jump V"() -> (w907:bool)
                      n414 = local read "V END"() -> (w906:i16)
                      n415 = case shown="True" w907 {
                        tunnel: w906 -> [w918 w919]
                        tunnel: [w917 w919] -> w905
                        tunnel: w909 -> [w916 _]
                        tunnel: [w915 TRUE ("Finished Move")] -> w908
                        frame False {
                          n416 = local read "ExpandVelScaller V"() -> (w910:i16)
                          n417 = local read "V VEl"() -> (w913:i16)
                          n418 = local read "V START"() -> (w914:i16)
                          n419 = Number To Boolean Array(number=w913) -> (Boolean array=w912:bool[])
                          n420 = Boolean Array To Number(Boolean array=w912) -> (number=w911:fxp<+/-,16,16>)
                          n421 = call "LinearMove.vi"("Time"=w916, "Start"=w914, "End"=w918, "Velocity"=w911, "ExpandVelScaller"=w910) -> ("OutPosition"=w917:i16, "Finished Move"=w915:bool)  [unwired: 13 in]
                        }
                        frame True {
                        }
                      }
                      n422 = local write "Applied Voltage"(w905) -> ()
                      n423 = xnode "FPGA I/O Node"("Connector0/AO3"=w905) -> ()  [unwired: 1 in, 1 out]
                    }
                    frame True {
                      n424 = local write "Applied Voltage"("V on Fly") -> ()
                      n425 = xnode "FPGA I/O Node"("Connector0/AO3"="V on Fly") -> ()  [unwired: 1 in, 1 out]
                    }
                  }
                }
                frame #2 {
                  n426 = local read "OnlyStopLineONCE V"() -> (w925:bool)
                  n427 = case shown="False" w925 {
                    tunnel: [w930 FALSE ("EndCurrentLine")] -> w926
                    frame False {
                      n428 = local read "EndCurrentLine"() -> (w930:bool)
                      n429 = case shown="True" w930 {
                        frame False {
                        }
                        frame True {
                          n430 = local write "OnlyStopLineONCE V"(TRUE ("EndCurrentLine")) -> ()
                        }
                      }
                    }
                    frame True {
                    }
                  }
                  n431 = local read "External Stop"() -> (w927:bool)
                  n432 = Or(x=w923, y=w926) -> (x .or. y?=w928:bool)
                  n433 = Or(x=w927, y=w928) -> (x .or. y?=w924:bool)
                }
              }
              n434 = local write "StopMoveV"(w872) -> ()
            }
          }
          frame True {
          }
        }
        n435 = case shown="False" w218 {
          tunnel: w213 -> [w818 _]
          frame False {
            n436 = while {
              shift-right: [w820] -> _
              shift-left: w818 -> [w823]
              stop <- w819 stop-if-true
              n437 = flat-sequence {
                tunnel: w823 -> [w825]
                tunnel: [w826] -> w824
                tunnel: w824 -> [w860]
                tunnel: [w860] -> w822
                tunnel: [w857] -> w821
                tunnel: [w867] -> w820
                tunnel: w822 -> [w867]
                tunnel: w821 -> [w861]
                tunnel: [w862] -> w819
                frame #0 {
                  n438 = local read "Internal Pause"() -> (w828:bool)
                  n439 = local read "External Pause"() -> (w829:bool)
                  n440 = Or(x=w829, y=w828) -> (x .or. y?=w827:bool)
                  n441 = case shown="True" w827 {
                    tunnel: w825 -> [w830 w833]
                    tunnel: [w830 w831] -> w826
                    frame False {
                    }
                    frame True {
                      n442 = global read "Tick Count.vi" "Tick Count"() -> (w832:u64)
                      n443 = while {
                        shift-right: [w845] -> w831
                        shift-left: w833 -> [w837]
                        shift-right: [w840] -> _
                        shift-left: w832 -> [w839]
                        stop <- w834 stop-if-true
                        n444 = local read "External Pause"() -> (w844:bool)
                        n445 = local read "Internal Pause"() -> (w842:bool)
                        n446 = global read "Tick Count.vi" "Tick Count"() -> (w840:u64)
                        n447 = local read "External Stop"() -> (w836:bool)
                        n448 = Not(x=w844) -> (.not. x?=w843:bool)
                        n449 = Not(x=w842) -> (.not. x?=w841:bool)
                        n450 = Subtract(x=w840, y=w839) -> (x-y=w838:u64)
                        n451 = And(x=w843, y=w841) -> (x .and. y?=w835:bool)
                        n452 = Add(x=w838, y=w837) -> (x+y=w845:u64)
                        n453 = Or(x=w835, y=w836) -> (x .or. y?=w834:bool)
                      }
                    }
                  }
                }
                frame #1 {
                  # "MAE 18/8/2014: Changed 0 to -32768 to allow -10 to 10V option. Note: as this is the full range of an I16 the coercion isn't doing much. In future make this boolean controlled from the T/F in advanced settings"
                  n454 = global read "Tick Count.vi" "Tick Count"() -> (w859:u64)
                  n455 = Subtract(x=w859, y=w860) -> (x-y=w846:u64)
                  n456 = To Fixed-Point(number=w846) -> (fixed-point=w858:fxp<+,64,64>)  [unwired: 1 in]
                  n457 = local read "X VEL"() -> (w850:i16)
                  n458 = local read "ExpandVelScaller X"() -> (w847:i16)
                  n459 = local read "X END"() -> (w848:i16)
                  n460 = local read "X START"() -> (w849:i16)
                  n461 = Number To Boolean Array(number=w850) -> (Boolean array=w856:bool[])
                  n462 = Boolean Array To Number(Boolean array=w856) -> (number=w855:fxp<+/-,16,16>)
                  n463 = call "LinearMove.vi"("Time"=w858, "Start"=w849, "End"=w848, "Velocity"=w855, "ExpandVelScaller"=w847) -> ("OutPosition"=w851:i16, "Finished Move"=w857:bool)  [unwired: 13 in]
                  n464 = In Range and Coerce(upper limit=i16 32767, x=w851, lower limit=i16 -32768) -> (coerced(x)=w852:i16)  [unwired: 1 out]
                  n465 = local write "Applied X"(w852) -> ()
                  n466 = xnode "I/O Node"("Connector0/AO0"=w852) -> ()  [unwired: 1 in, 1 out]
                }
                frame #2 {
                  n467 = local read "OnlyStopLineONCE X"() -> (w864:bool)
                  n468 = case shown="False" w864 {
                    tunnel: [w868 FALSE ("EndCurrentLine")] -> w863
                    frame False {
                      n469 = local read "EndCurrentLine"() -> (w868:bool)
                      n470 = case shown="True" w868 {
                        frame False {
                        }
                        frame True {
                          n471 = local write "OnlyStopLineONCE X"(TRUE ("EndCurrentLine")) -> ()
                        }
                      }
                    }
                    frame True {
                    }
                  }
                  n472 = local read "External Stop"() -> (w866:bool)
                  n473 = Or(x=w861, y=w863) -> (x .or. y?=w865:bool)
                  n474 = Or(x=w866, y=w865) -> (x .or. y?=w862:bool)
                }
              }
              n475 = local write "StopMoveX"(w819) -> ()
            }
          }
          frame True {
          }
        }
        n476 = case shown="False" w217 {
          tunnel: w213 -> [w765 _]
          frame False {
            n477 = while {
              shift-right: [w767] -> _
              shift-left: w765 -> [w770]
              stop <- w766 stop-if-true
              n478 = flat-sequence {
                tunnel: w770 -> [w772]
                tunnel: [w773] -> w771
                tunnel: w771 -> [w807]
                tunnel: [w807] -> w769
                tunnel: [w804] -> w768
                tunnel: [w814] -> w767
                tunnel: w769 -> [w814]
                tunnel: w768 -> [w808]
                tunnel: [w809] -> w766
                frame #0 {
                  n479 = local read "External Pause"() -> (w776:bool)
                  n480 = local read "Internal Pause"() -> (w775:bool)
                  n481 = Or(x=w776, y=w775) -> (x .or. y?=w774:bool)
                  n482 = case shown="True" w774 {
                    tunnel: w772 -> [w777 w780]
                    tunnel: [w777 w778] -> w773
                    frame False {
                    }
                    frame True {
                      n483 = global read "Tick Count.vi" "Tick Count"() -> (w779:u64)
                      n484 = while {
                        shift-right: [w792] -> w778
                        shift-left: w780 -> [w784]
                        shift-right: [w787] -> _
                        shift-left: w779 -> [w786]
                        stop <- w781 stop-if-true
                        n485 = local read "External Pause"() -> (w791:bool)
                        n486 = local read "Internal Pause"() -> (w789:bool)
                        n487 = global read "Tick Count.vi" "Tick Count"() -> (w787:u64)
                        n488 = local read "External Stop"() -> (w783:bool)
                        n489 = Not(x=w791) -> (.not. x?=w790:bool)
                        n490 = Not(x=w789) -> (.not. x?=w788:bool)
                        n491 = Subtract(x=w787, y=w786) -> (x-y=w785:u64)
                        n492 = And(x=w790, y=w788) -> (x .and. y?=w782:bool)
                        n493 = Add(x=w785, y=w784) -> (x+y=w792:u64)
                        n494 = Or(x=w782, y=w783) -> (x .or. y?=w781:bool)
                      }
                    }
                  }
                }
                frame #1 {
                  # "MAE 18/8/2014: Changed 0 to -32768 to allow -10 to 10V option. Note: as this is the full range of an I16 the coercion isn't doing much. In future make this boolean controlled from the T/F in advanced settings"
                  n495 = global read "Tick Count.vi" "Tick Count"() -> (w806:u64)
                  n496 = Subtract(x=w806, y=w807) -> (x-y=w793:u64)
                  n497 = To Fixed-Point(number=w793) -> (fixed-point=w805:fxp<+,64,64>)  [unwired: 1 in]
                  n498 = local read "Y VEL"() -> (w797:i16)
                  n499 = local read "ExpandVelScaller Y"() -> (w794:i16)
                  n500 = local read "Y END"() -> (w795:i16)
                  n501 = local read "Y START"() -> (w796:i16)
                  n502 = Number To Boolean Array(number=w797) -> (Boolean array=w803:bool[])
                  n503 = Boolean Array To Number(Boolean array=w803) -> (number=w802:fxp<+/-,16,16>)
                  n504 = call "LinearMove.vi"("Time"=w805, "Start"=w796, "End"=w795, "Velocity"=w802, "ExpandVelScaller"=w794) -> ("OutPosition"=w798:i16, "Finished Move"=w804:bool)  [unwired: 13 in]
                  n505 = In Range and Coerce(upper limit=i16 32767, x=w798, lower limit=i16 -32768) -> (coerced(x)=w799:i16)  [unwired: 1 out]
                  n506 = local write "Applied Y"(w799) -> ()
                  n507 = xnode "I/O Node"("Connector0/AO1"=w799) -> ()  [unwired: 1 in, 1 out]
                }
                frame #2 {
                  n508 = local read "OnlyStopLineONCE Y"() -> (w810:bool)
                  n509 = case shown="False" w810 {
                    tunnel: [w815 FALSE ("EndCurrentLine")] -> w811
                    frame False {
                      n510 = local read "EndCurrentLine"() -> (w815:bool)
                      n511 = case shown="True" w815 {
                        frame False {
                        }
                        frame True {
                          n512 = local write "OnlyStopLineONCE Y"(TRUE ("EndCurrentLine")) -> ()
                        }
                      }
                    }
                    frame True {
                    }
                  }
                  n513 = local read "External Stop"() -> (w813:bool)
                  n514 = Or(x=w808, y=w811) -> (x .or. y?=w812:bool)
                  n515 = Or(x=w813, y=w812) -> (x .or. y?=w809:bool)
                }
              }
              n516 = local write "StopMoveY"(w766) -> ()
            }
          }
          frame True {
          }
        }
        n517 = case shown="False" w216 {
          tunnel: w213 -> [w355 _]
          frame False {
            n518 = local read "Applied X"() -> (w354:i16)
            n519 = while {
              shift-right: [w359] -> _
              shift-left: w355 -> [w362]
              shift-right: [w356] -> _
              shift-left: w354 -> [w357]
              stop <- w358 stop-if-true
              n520 = flat-sequence {
                tunnel: w362 -> [w365]
                tunnel: [w366] -> w363
                tunnel: w363 -> [w403]
                tunnel: [w403] -> w361
                tunnel: [w398] -> w360
                tunnel: w357 -> [w392]
                tunnel: [w391] -> w356
                tunnel: [w761] -> w359
                tunnel: w361 -> [w761]
                tunnel: w360 -> [w755]
                tunnel: [w756] -> w358
                frame #0 {
                  n521 = local read "Update Position Loop Wait Time (ms)"() -> (w364:u16)
                  n522 = local read "External Pause"() -> (w369:bool)
                  n523 = local read "Internal Pause"() -> (w368:bool)
                  n524 = Or(x=w369, y=w368) -> (x .or. y?=w367:bool)
                  n525 = case shown="True" w367 {
                    tunnel: w365 -> [w370 w373]
                    tunnel: [w370 w371] -> w366
                    frame False {
                    }
                    frame True {
                      n526 = global read "Tick Count.vi" "Tick Count"() -> (w372:u64)
                      n527 = while {
                        shift-right: [w385] -> w371
                        shift-left: w373 -> [w377]
                        shift-right: [w380] -> _
                        shift-left: w372 -> [w379]
                        stop <- w374 stop-if-true
                        n528 = local read "External Pause"() -> (w384:bool)
                        n529 = local read "Internal Pause"() -> (w382:bool)
                        n530 = global read "Tick Count.vi" "Tick Count"() -> (w380:u64)
                        n531 = local read "External Stop"() -> (w376:bool)
                        n532 = Not(x=w384) -> (.not. x?=w383:bool)
                        n533 = Not(x=w382) -> (.not. x?=w381:bool)
                        n534 = Subtract(x=w380, y=w379) -> (x-y=w378:u64)
                        n535 = And(x=w383, y=w381) -> (x .and. y?=w375:bool)
                        n536 = Add(x=w378, y=w377) -> (x+y=w385:u64)
                        n537 = Or(x=w375, y=w376) -> (x .or. y?=w374:bool)
                      }
                    }
                  }
                  n538 = call "Loop Timer"("Count(mSec)"=w364) -> ()  [unwired: 1 out]
                }
                frame #1 {
                  # "MAE 18/8/2014: Changed 0 to -32768 to allow -10 to 10V option. Note: as this is the full range of an I16 the coercion isn't doing much. In future make this boolean controlled from the T/F in advanced settings"
                  n539 = global read "Tick Count.vi" "Tick Count"() -> (w402:u64)
                  n540 = local read "Feedback2 Boolean"() -> (w386:bool)
                  n541 = local read "LineType"() -> (w389:i16)
                  n542 = local read "Feedback1 Boolean"() -> (w387:bool)
                  n543 = Subtract(x=w402, y=w403) -> (x-y=w394:u64)
                  n544 = To Fixed-Point(number=w394) -> (fixed-point=w390:fxp<+,64,64>)  [unwired: 1 in]
                  n545 = Or(x=w387, y=w386) -> (x .or. y?=w388:bool)
                  n546 = case shown="15" w389 {
                    tunnel: "P" -> [_ _ _ w439 w451 w467 w488 _ w523 _ _ _ _]
                    tunnel: [w406 w416 w423 w434 w447 w462 w478 w511 w518 w540 w605 w678 w741] -> w398
                    tunnel: [w405 w415 w425 w437 w449 w465 w477 w514 w521 w542 w607 w680 w746] -> w397
                    tunnel: "Upper limit Of dZ" -> [_ _ _ w433 w448 w464 w487 _ w517 _ _ _ _]
                    tunnel: w392 -> [_ _ _ _ _ _ w485 _ _ _ _ _ _]
                    tunnel: [_ _ _ _ _ _ w484 _ _ _ _ _ _] -> w391
                    tunnel: w390 -> [w404 w414 w424 _ _ _ _ _ _ w541 w606 w679 _]
                    tunnel: w388 -> [_ w413 w423 _ _ _ _ _ _ _ _ _ _]
                    tunnel: w386 -> [_ _ _ _ _ _ _ _ w516 _ _ _ _]
                    frame 0, Default {
                      # "Normal Move"
                      n547 = local read "Z VEL"() -> (w409:i16)
                      n548 = local read "ExpandVelScaller Z"() -> (w412:i16)
                      n549 = local read "Z END"() -> (w411:i16)
                      n550 = local read "Z START"() -> (w410:i16)
                      n551 = Number To Boolean Array(number=w409) -> (Boolean array=w407:bool[])
                      n552 = Boolean Array To Number(Boolean array=w407) -> (number=w408:fxp<+/-,16,16>)
                      n553 = call "LinearMove.vi"("Time"=w404, "Start"=w410, "End"=w411, "Velocity"=w408, "ExpandVelScaller"=w412) -> ("OutPosition"=w405:i16, "Finished Move"=w406:bool)  [unwired: 13 in]
                    }
                    frame 1 {
                      # "Pause on Set Point"
                      n554 = local write "Internal Pause"(w413) -> ()
                      n555 = local read "Z VEL"() -> (w419:i16)
                      n556 = local read "ExpandVelScaller Z"() -> (w422:i16)
                      n557 = local read "Z END"() -> (w421:i16)
                      n558 = local read "Z START"() -> (w420:i16)
                      n559 = Number To Boolean Array(number=w419) -> (Boolean array=w417:bool[])
                      n560 = Boolean Array To Number(Boolean array=w417) -> (number=w418:fxp<+/-,16,16>)
                      n561 = call "LinearMove.vi"("Time"=w414, "Start"=w420, "End"=w421, "Velocity"=w418, "ExpandVelScaller"=w422) -> ("OutPosition"=w415:i16, "Finished Move"=w416:bool)  [unwired: 13 in]
                    }
                    frame 2 {
                      # "STOP Current Move on SetPoint"
                      n562 = local read "Z VEL"() -> (w428:i16)
                      n563 = local read "ExpandVelScaller Z"() -> (w431:i16)
                      n564 = local read "Z END"() -> (w430:i16)
                      n565 = local read "Z START"() -> (w429:i16)
                      n566 = Number To Boolean Array(number=w428) -> (Boolean array=w426:bool[])
                      n567 = Boolean Array To Number(Boolean array=w426) -> (number=w427:fxp<+/-,16,16>)
                      n568 = call "LinearMove.vi"("Time"=w424, "Start"=w429, "End"=w430, "Velocity"=w427, "ExpandVelScaller"=w431) -> ("OutPosition"=w425:i16)  [unwired: 13 in, 1 out]
                    }
                    frame 4 {
                      # "For scanning-Propotional Controller for constant distance scanning"
                      n569 = local read "Feedback1 Error"() -> (w432:i32)
                      n570 = Multiply(x=w439, y=w432) -> (x*y=w444:fxp<+/-,64,33>)
                      n571 = To Word Integer(number=w444) -> (16bit integer=w443:i16)
                      n572 = To Long Integer(number=w443) -> (32bit integer=w445:i32)
                      n573 = local read "StopMoveY"() -> (w435:bool)
                      n574 = local read "StopMoveX"() -> (w436:bool)
                      n575 = local read "Applied Z"() -> (w438:i16)
                      n576 = Negate(x=w433) -> (-x=w440:i32)
                      n577 = And(x=w436, y=w435) -> (x .and. y?=w434:bool)
                      n578 = In Range and Coerce(upper limit=w433, x=w445, lower limit=w440) -> (coerced(x)=w441:i32)  [unwired: 1 out]
                      n579 = To Long Integer(number=w438) -> (32bit integer=w442:i32)
                      n580 = Add(x=w442, y=w441) -> (x+y=w437:i32)
                    }
                    frame 11 {
                      # "Dependent on hold time-Propotional Controller for constant distance scanning"
                      n581 = local read "Feedback1 Error"() -> (w446:i32)
                      n582 = Multiply(x=w451, y=w446) -> (x*y=w456:fxp<+/-,64,33>)
                      n583 = To Word Integer(number=w456) -> (16bit integer=w455:i16)
                      n584 = To Long Integer(number=w455) -> (32bit integer=w457:i32)
                      n585 = local read "HasHeldHoldTimeHappend?"() -> (w447:bool)
                      n586 = local read "Applied Z"() -> (w450:i16)
                      n587 = Negate(x=w448) -> (-x=w452:i32)
                      n588 = In Range and Coerce(upper limit=w448, x=w457, lower limit=w452) -> (coerced(x)=w453:i32)  [unwired: 1 out]
                      n589 = To Long Integer(number=w450) -> (32bit integer=w454:i32)
                      n590 = Add(x=w454, y=w453) -> (x+y=w449:i32)
                    }
                    frame 10 {
                      # "deciding the limit of the Z movement (up or down) regardless of the x value"
                      # "convert the difference in siganls to distance in um"
                      # "External signal-Feedback_Threshold"
                      # "Dependent on holdtime-Propotional Controller for constant distance scanning ONLY for POSITIVE"
                      n591 = local read "Feedback1 Error"() -> (w458:i32)
                      n592 = Multiply(x=w467, y=w458) -> (x*y=w471:fxp<+/-,64,33>)
                      n593 = To Word Integer(number=w471) -> (16bit integer=w470:i16)
                      n594 = To Long Integer(number=w470) -> (32bit integer=w472:i32)
                      n595 = Negate(x=w464) -> (-x=w468:i32)
                      n596 = In Range and Coerce(upper limit=w464, x=w472, lower limit=w468) -> (coerced(x)=w460:i32)  [unwired: 1 out]
                      n597 = Less?(x=w460, y=0) -> (x < y?=w461:bool)
                      n598 = local read "HasHeldHoldTimeHappend?"() -> (w462:bool)
                      n599 = case shown="True" w461 {
                        tunnel: w460 -> [_ w474]
                        tunnel: [0 w474] -> w463
                        frame False {
                        }
                        frame True {
                        }
                      }
                      n600 = local read "Applied Z"() -> (w466:i16)
                      n601 = To Long Integer(number=w466) -> (32bit integer=w469:i32)
                      n602 = Add(x=w469, y=w463) -> (x+y=w465:i32)
                    }
                    frame 5 {
                      # "Proportional controller for constant distance scanning - with storing the positions in a buffer"
                      n603 = local read "Feedback1 Error"() -> (w475:i32)
                      n604 = local read "TraceRetraceFirstUse"() -> (w476:bool)
                      n605 = local read "Applied X"() -> (w484:i16)
                      n606 = local read "Applied Z"() -> (w486:i16)
                      n607 = Multiply(x=w488, y=w475) -> (x*y=w490:fxp<+/-,64,33>)
                      n608 = To Word Integer(number=w490) -> (16bit integer=w491:i16)
                      n609 = Subtract(x=w484, y=w485) -> (x-y=w483:i16)
                      n610 = To Long Integer(number=w491) -> (32bit integer=w489:i32)
                      n611 = case shown="False" w476 {
                        tunnel: w483 -> [w503 w506]
                        tunnel: [w502 w506] -> w482
                        tunnel: [w501 w505] -> w481
                        tunnel: w485 -> [w501 w504]
                        frame False {
                          n612 = Increment(x=w503) -> (x+1=w502:i16)
                        }
                        frame True {
                          n613 = Increment(x=w504) -> (x+1=w505:i16)
                        }
                      }
                      n614 = Negate(x=w487) -> (-x=w494:i32)
                      n615 = In Range and Coerce(upper limit=w487, x=w489, lower limit=w494) -> (coerced(x)=w493:i32)  [unwired: 1 out]
                      n616 = To Long Integer(number=w486) -> (32bit integer=w492:i32)
                      n617 = Add(x=w492, y=w493) -> (x+y=w477:i32)
                      n618 = for {
                        N: w482 -> [_]
                        shift-right: [w496] -> _
                        shift-left: w481 -> [w497]
                        tunnel: w477 -> [w500]
                        n619 = To Unsigned Long Integer(number=w497) -> (unsigned 32bit integer=w498:u32)
                        n620 = To Word Integer(number=w500) -> (16bit integer=w499:i16)
                        n621 = local write "TraceRetraceFirstUse"(TRUE ("TraceRetraceFirst?")) -> ()
                        n622 = xnode ("Memory Write")("Address"=w498, "Data"=w499) -> ()  [unwired: 1 in, 1 out]
                        n623 = Increment(x=w497) -> (x+1=w496:i16)
                      }
                      n624 = local read "StopMoveY"() -> (w479:bool)
                      n625 = local read "StopMoveX"() -> (w480:bool)
                      n626 = And(x=w480, y=w479) -> (x .and. y?=w478:bool)
                    }
                    frame 6 {
                      # "retrace the Z positions stored in the buffer, see feedbaack type 5"
                      n627 = local read "Applied X"() -> (w507:i16)
                      n628 = To Unsigned Long Integer(number=w507) -> (unsigned 32bit integer=w510:u32)
                      n629 = Add(x="Xoffset", y=w510) -> (x+y=w508:u32)
                      n630 = xnode ("Memory Read")("Address"=w508) -> ("Data"=w514:i16)  [unwired: 1 in, 1 out]
                      n631 = local read "StopMoveY"() -> (w512:bool)
                      n632 = local read "StopMoveX"() -> (w513:bool)
                      n633 = And(x=w513, y=w512) -> (x .and. y?=w511:bool)
                    }
                    frame 7 {
                      # "Proportianal controller for constant distance scan, with ability to pause based on a secondary signal"
                      n634 = local write "Internal Pause"(w516) -> ()
                      n635 = local read "Feedback1 Error"() -> (w515:i32)
                      n636 = Multiply(x=w523, y=w515) -> (x*y=w528:fxp<+/-,64,33>)
                      n637 = To Word Integer(number=w528) -> (16bit integer=w527:i16)
                      n638 = To Long Integer(number=w527) -> (32bit integer=w529:i32)
                      n639 = local read "StopMoveY"() -> (w519:bool)
                      n640 = local read "StopMoveX"() -> (w520:bool)
                      n641 = local read "Applied Z"() -> (w522:i16)
                      n642 = Negate(x=w517) -> (-x=w524:i32)
                      n643 = And(x=w520, y=w519) -> (x .and. y?=w518:bool)
                      n644 = In Range and Coerce(upper limit=w517, x=w529, lower limit=w524) -> (coerced(x)=w525:i32)  [unwired: 1 out]
                      n645 = To Long Integer(number=w522) -> (32bit integer=w526:i32)
                      n646 = Add(x=w526, y=w525) -> (x+y=w521:i32)
                    }
                    frame 8 {
                      # "Sum of most recent 1024"
                      n647 = local read "FeedBackType"() -> (w532:u8)
                      n648 = local read "Count Average"() -> (w533:i16)
                      n649 = case shown="1" w532 {
                        tunnel: [w545 w546 w547 w548 w549 w550] -> w531
                        frame 0, Default {
                          n650 = local read "Ext amp"() -> (w545:i16)
                        }
                        frame 1 {
                          n651 = local read "MeasuredCurrent"() -> (w546:i16)
                        }
                        frame 2 {
                          n652 = local read "MeasuredCurrent 2"() -> (w547:i16)
                        }
                        frame 3 {
                          n653 = local read "Ext Phase"() -> (w548:i16)
                        }
                        frame 4 {
                          n654 = local read "MeasuredCurrent"() -> (w549:i16)
                        }
                        frame 5 {
                          n655 = local read "MeasuredCurrent 2"() -> (w550:i16)
                        }
                      }
                      n656 = Equal?(x=w533, y="P2AvgWhole") -> (x = y?=w543:bool)
                      n657 = local read "ExtraTime 2"() -> (w536:fxp<+,64,64>)
                      n658 = To Long Integer(number=w531) -> (32bit integer=w530:i32)
                      n659 = local read "AverageSum"() -> (w539:i64)
                      n660 = case shown="True" w543 {
                        tunnel: w530 -> [w559 w580]
                        tunnel: w539 -> [w560 w587]
                        tunnel: [w561 w587] -> w544
                        tunnel: w533 -> [w558 w574]
                        tunnel: [w557 w574] -> w538
                        tunnel: [w556 w588] -> w542
                        tunnel: w541 -> [w554 w582]
                        tunnel: [FALSE w576] -> w540
                        tunnel: [w554 w584] -> w537
                        tunnel: w536 -> [_ w584]
                        tunnel: [w551 w572] -> w535
                        frame False {
                          n661 = local read "SampleIterator"() -> (w551:i16)
                          n662 = local read "IterateHolder"() -> (w553:i16)
                          n663 = Less?(x=w551, y=w553) -> (x < y?=w552:bool)
                          n664 = case shown="True" w552 {
                            tunnel: [w562 w569] -> w561
                            tunnel: w560 -> [w562 w568]
                            tunnel: w559 -> [_ w564]
                            tunnel: w558 -> [w563 w566]
                            tunnel: [w563 w567] -> w557
                            frame False {
                            }
                            frame True {
                              # "Count up to 1024 (start at 0) data points then start moving"
                              n665 = To Quad Integer(1:w564) -> (0:w565:i64)
                              n666 = Increment(x=w566) -> (x+1=w567:i16)
                              n667 = Add(x=w568, y=w565) -> (x+y=w569:i64)
                            }
                          }
                          n668 = local read "Applied Z"() -> (w556:i16)
                        }
                        frame True {
                          # "STOP Current Move on SetPoint"
                          n669 = local read "AverageSum"() -> (w586:i64)
                          n670 = local read "Feedback_Threshold"() -> (w571:i64)
                          n671 = Subtract(x=w582, y=w584) -> (x-y=w585:fxp<+/-,64,65>)
                          n672 = Scale By Power Of 2(n="P2AvgMinus", x=w586) -> (x*2^n=w575:i64)
                          n673 = To Fixed-Point(fixed-point type=w582, number=w585) -> (fixed-point=w583:fxp<+,64,64>)
                          n674 = To Long Integer(number=w571) -> (32bit integer=w570:i32)
                          n675 = local read "Z VEL"() -> (w591:i16)
                          n676 = Subtract(x=w575, y=w570) -> (x-y=w581:i64)
                          n677 = local read "ExpandVelScaller Z"() -> (w594:i16)
                          n678 = local read "Z END"() -> (w593:i16)
                          n679 = local read "Z START"() -> (w592:i16)
                          n680 = Number To Boolean Array(number=w591) -> (Boolean array=w589:bool[])
                          n681 = Add(x=w570, y=w575) -> (x+y=w579:i64)
                          n682 = Boolean Array To Number(Boolean array=w589) -> (number=w590:fxp<+/-,16,16>)
                          n683 = Greater?(x=w580, y=w579) -> (0:w578:bool)
                          n684 = call "LinearMove.vi"("Time"=w583, "Start"=w592, "End"=w593, "Velocity"=w590, "ExpandVelScaller"=w594) -> ("OutPosition"=w588:i16)  [unwired: 13 in, 1 out]
                          n685 = Less?(x=w580, y=w581) -> (x < y?=w577:bool)
                          n686 = Or(x=w578, y=w577) -> (x .or. y?=w576:bool)
                          n687 = local read "SampleNum"() -> (w572:i16)
                        }
                      }
                      "ExtraTime 2" <- w537
                      n688 = local write "IterateHolder"(w535) -> ()
                      n689 = local write "AverageSum"(w544) -> ()
                      n690 = local write "Count Average"(w538) -> ()
                    }
                    frame 9 {
                      # "Sum of most recent 1024"
                      n691 = local read "FeedBackType"() -> (w597:u8)
                      n692 = local read "P2AvgWhole"() -> (w598:i32)
                      n693 = local read "Count Average"() -> (w602:i16)
                      n694 = case shown="1" w597 {
                        tunnel: [w610 w611 w612 w613 w614 w615] -> w596
                        frame 0, Default {
                          n695 = local read "Ext amp"() -> (w610:i16)
                        }
                        frame 1 {
                          n696 = local read "MeasuredCurrent"() -> (w611:i16)
                        }
                        frame 2 {
                          n697 = local read "MeasuredCurrent 2"() -> (w612:i16)
                        }
                        frame 3 {
                          n698 = local read "Ext Phase"() -> (w613:i16)
                        }
                        frame 4 {
                          n699 = local read "MeasuredCurrent"() -> (w614:i16)
                        }
                        frame 5 {
                          n700 = local read "MeasuredCurrent 2"() -> (w615:i16)
                        }
                      }
                      n701 = Equal?(x=w602, y=w598) -> (x = y?=w608:bool)
                      n702 = local read "ExtraTime 3"() -> (w600:fxp<+,64,64>)
                      n703 = To Long Integer(number=w596) -> (32bit integer=w595:i32)
                      n704 = local read "AverageSum"() -> (w604:i64)
                      n705 = case shown="True" w608 {
                        tunnel: w595 -> [w624 w637]
                        tunnel: w604 -> [w625 _]
                        tunnel: [w626 w639] -> w609
                        tunnel: w602 -> [w623 w645]
                        tunnel: [w622 w645] -> w603
                        tunnel: [w621 w655] -> w607
                        tunnel: w606 -> [w619 w651]
                        tunnel: [FALSE w646] -> w605
                        tunnel: [w619 w653] -> w601
                        tunnel: w600 -> [_ w653]
                        tunnel: [w616 w642] -> w599
                        frame False {
                          n706 = local read "SampleIterator"() -> (w616:i16)
                          n707 = local read "IterateHolder"() -> (w618:i16)
                          n708 = Less?(x=w616, y=w618) -> (x < y?=w617:bool)
                          n709 = case shown="True" w617 {
                            tunnel: [w627 w634] -> w626
                            tunnel: w625 -> [w627 w633]
                            tunnel: w624 -> [_ w632]
                            tunnel: w623 -> [w628 w630]
                            tunnel: [w628 w629] -> w622
                            frame False {
                            }
                            frame True {
                              # "Count up to 1024 (start at 0) data points then start moving"
                              n710 = To Quad Integer(1:w632) -> (0:w631:i64)
                              n711 = Increment(x=w630) -> (x+1=w629:i16)
                              n712 = Add(x=w633, y=w631) -> (x+y=w634:i64)
                            }
                          }
                          n713 = local read "Applied Z"() -> (w621:i16)
                        }
                        frame True {
                          # "STOP Current Move on SetPoint"
                          n714 = local read "AverageSum"() -> (w641:i64)
                          n715 = local read "P2AvgMinus"() -> (w638:i32)
                          n716 = local read "Feedback_Threshold"() -> (w636:i64)
                          n717 = To Long Integer(number=w636) -> (32bit integer=w635:i32)
                          n718 = Subtract(x=w651, y=w653) -> (x-y=w654:fxp<+/-,64,65>)
                          n719 = Scale By Power Of 2(n=w638, x=w641) -> (x*2^n=w640:i64)
                          n720 = Subtract(x=w640, y=w635) -> (x-y=w650:i64)
                          n721 = local read "SampleIterator"() -> (w642:i16)
                          n722 = To Fixed-Point(fixed-point type=w651, number=w654) -> (fixed-point=w652:fxp<+,64,64>)
                          n723 = local read "IterateHolder"() -> (w644:i16)
                          n724 = Add(x=w635, y=w640) -> (x+y=w649:i64)
                          n725 = local read "Z VEL"() -> (w658:i16)
                          n726 = Less?(x=w642, y=w644) -> (x < y?=w643:bool)
                          "x < y?" <- w643
                          n727 = Greater?(x=w637, y=w649) -> (0:w648:bool)
                          n728 = local read "ExpandVelScaller Z"() -> (w661:i16)
                          n729 = local read "Z END"() -> (w660:i16)
                          n730 = Less?(x=w637, y=w650) -> (x < y?=w647:bool)
                          n731 = local read "Z START"() -> (w659:i16)
                          n732 = Or(x=w648, y=w647) -> (x .or. y?=w646:bool)
                          n733 = Number To Boolean Array(number=w658) -> (Boolean array=w656:bool[])
                          n734 = Boolean Array To Number(Boolean array=w656) -> (number=w657:fxp<+/-,16,16>)
                          n735 = call "LinearMove.vi"("Time"=w652, "Start"=w659, "End"=w660, "Velocity"=w657, "ExpandVelScaller"=w661) -> ("OutPosition"=w655:i16)  [unwired: 13 in, 1 out]
                          n736 = case shown="True" w643 {
                            tunnel: w641 -> [w662 w667]
                            tunnel: w640 -> [_ w666]
                            tunnel: [w662 w664] -> w639
                            tunnel: w637 -> [_ w663]
                            frame False {
                            }
                            frame True {
                              n737 = Subtract(x=w667, y=w666) -> (x-y=w665:i64)
                              n738 = Add(x=w665, y=w663) -> (x+y=w664:i64)
                            }
                          }
                        }
                      }
                      "ExtraTime 3" <- w601
                      n739 = local write "IterateHolder"(w599) -> ()
                      n740 = local write "AverageSum"(w609) -> ()
                      n741 = local write "Count Average"(w603) -> ()
                    }
                    frame 14 {
                      # "Sum of most recent 1024"
                      n742 = local read "FeedBackType"() -> (w670:u8)
                      n743 = local read "Count Average"() -> (w672:i16)
                      n744 = local read "P2AvgWhole"() -> (w671:i32)
                      n745 = case shown="1" w670 {
                        tunnel: [w683 w684 w685 w686 w687 w688] -> w669
                        frame 0, Default {
                          n746 = local read "Ext amp"() -> (w683:i16)
                        }
                        frame 1 {
                          n747 = local read "MeasuredCurrent"() -> (w684:i16)
                        }
                        frame 2 {
                          n748 = local read "MeasuredCurrent 2"() -> (w685:i16)
                        }
                        frame 3 {
                          n749 = local read "Ext Phase"() -> (w686:i16)
                        }
                        frame 4 {
                          n750 = local read "MeasuredCurrent"() -> (w687:i16)
                        }
                        frame 5 {
                          n751 = local read "MeasuredCurrent 2"() -> (w688:i16)
                        }
                      }
                      n752 = Equal?(x=w672, y=w671) -> (x = y?=w681:bool)
                      n753 = local read "ExtraTime 4"() -> (w674:fxp<+,64,64>)
                      n754 = To Long Integer(number=w669) -> (32bit integer=w668:i32)
                      n755 = local read "AverageSum"() -> (w677:i64)
                      n756 = case shown="True" w681 {
                        tunnel: w668 -> [w697 w726]
                        tunnel: w677 -> [w698 w732]
                        tunnel: [w699 w732] -> w682
                        tunnel: w672 -> [w696 w722]
                        tunnel: [w695 w722] -> w676
                        tunnel: [w694 w733] -> w680
                        tunnel: w679 -> [w692 w727]
                        tunnel: [FALSE w723] -> w678
                        tunnel: [w692 w729] -> w675
                        tunnel: w674 -> [_ w729]
                        tunnel: [w689 w721] -> w673
                        frame False {
                          n757 = local read "SampleIterator"() -> (w689:i16)
                          n758 = local read "IterateHolder"() -> (w691:i16)
                          n759 = Less?(x=w689, y=w691) -> (x < y?=w690:bool)
                          n760 = case shown="True" w690 {
                            tunnel: [w700 w707] -> w699
                            tunnel: w698 -> [w700 w706]
                            tunnel: w697 -> [_ w702]
                            tunnel: w696 -> [w701 w704]
                            tunnel: [w701 w705] -> w695
                            frame False {
                            }
                            frame True {
                              # "Count up to 1024 (start at 0) data points then start moving"
                              n761 = To Quad Integer(1:w702) -> (0:w703:i64)
                              n762 = Increment(x=w704) -> (x+1=w705:i16)
                              n763 = Add(x=w706, y=w703) -> (x+y=w707:i64)
                            }
                          }
                          n764 = local read "Applied Z"() -> (w694:i16)
                        }
                        frame True {
                          # "STOP Current Move on SetPoint"
                          n765 = local read "P2AvgMinus"() -> (w709:i32)
                          n766 = local read "Feedback_Threshold"() -> (w708:i64)
                          n767 = local read "AverageSum"() -> (w731:i64)
                          n768 = Subtract(x=w727, y=w729) -> (x-y=w730:fxp<+/-,64,65>)
                          n769 = To Quad Integer(1:w726) -> (0:w720:i64)
                          n770 = Scale By Power Of 2(n=w709, x=w731) -> (x*2^n=w716:i64)
                          n771 = To Fixed-Point(fixed-point type=w727, number=w730) -> (fixed-point=w728:fxp<+,64,64>)
                          n772 = To Quad Integer(1:w716) -> (0:w717:i64)
                          n773 = To Quad Integer(1:w708) -> (0:w712:i64)
                          n774 = Scale By Power Of 2(n=i16 15, x=w720) -> (x*2^n=w710:i64)
                          n775 = Scale By Power Of 2(n=i16 15, x=w717) -> (x*2^n=w711:i64)
                          n776 = local read "Z VEL"() -> (w736:i16)
                          n777 = local read "ExpandVelScaller Z"() -> (w739:i16)
                          n778 = Multiply(x=w716, y=w712) -> (x*y=w714:i64)
                          n779 = local read "Z END"() -> (w738:i16)
                          n780 = local read "Z START"() -> (w737:i16)
                          n781 = Number To Boolean Array(number=w736) -> (Boolean array=w734:bool[])
                          n782 = Add(x=w711, y=w714) -> (x+y=w715:i64)
                          n783 = Boolean Array To Number(Boolean array=w734) -> (number=w735:fxp<+/-,16,16>)
                          n784 = Subtract(x=w711, y=w714) -> (x-y=w713:i64)
                          n785 = Greater?(x=w710, y=w715) -> (0:w725:bool)
                          n786 = call "LinearMove.vi"("Time"=w728, "Start"=w737, "End"=w738, "Velocity"=w735, "ExpandVelScaller"=w739) -> ("OutPosition"=w733:i16)  [unwired: 13 in, 1 out]
                          n787 = Less?(x=w710, y=w713) -> (x < y?=w724:bool)
                          n788 = Or(x=w725, y=w724) -> (x .or. y?=w723:bool)
                          n789 = local read "SampleNum"() -> (w721:i16)
                        }
                      }
                      "ExtraTime 4" <- w675
                      n790 = local write "AverageSum"(w682) -> ()
                      n791 = local write "Count Average"(w676) -> ()
                      n792 = local write "IterateHolder"(w673) -> ()
                    }
                    frame 15 {
                      # "Charge accumulator\nKM 25/11/22"
                      n793 = local read "FeedBackType"() -> (w747:u8)
                      n794 = case shown="1" w747 {
                        tunnel: [w749 w750 w751 w752 w753 w754] -> w744
                        frame 0, Default {
                          n795 = local read "Ext amp"() -> (w749:i16)
                        }
                        frame 1 {
                          n796 = local read "MeasuredCurrent"() -> (w750:i16)
                        }
                        frame 2 {
                          n797 = local read "MeasuredCurrent 2"() -> (w751:i16)
                        }
                        frame 3 {
                          n798 = local read "Ext Phase"() -> (w752:i16)
                        }
                        frame 4 {
                          n799 = local read "MeasuredCurrent"() -> (w753:i16)
                        }
                        frame 5 {
                          n800 = local read "MeasuredCurrent 2"() -> (w754:i16)
                        }
                      }
                      n801 = local read "AverageSum"() -> (w748:i64)
                      n802 = local read "Feedback_Threshold 2"() -> (w740:i32)
                      n803 = To Quad Integer(1:w744) -> (0:w745:i64)
                      n804 = Add(x=w748, y=w745) -> (x+y=w743:i64)
                      n805 = local write "AverageSum"(w743) -> ()
                      n806 = Absolute Value(x=w743) -> (abs(x)=w742:i64)
                      n807 = Greater?(x=w742, y=w740) -> (0:w741:bool)
                      n808 = local read "Applied Z"() -> (w746:i16)
                    }
                  }
                  n809 = In Range and Coerce(upper limit=32767, x=w397, lower limit=-32768) -> (coerced(x)=w396:i32)  [unwired: 1 out]
                  n810 = To Word Integer(number=w396) -> (16bit integer=w395:i16)
                  n811 = xnode "I/O Node"("Connector0/AO2"=w395) -> ()  [unwired: 1 in, 1 out]
                  n812 = local write "Applied Z"(w395) -> ()
                }
                frame #2 {
                  n813 = local read "OnlyStopLineONCE Z"() -> (w758:bool)
                  n814 = case shown="True" w758 {
                    tunnel: [w762 FALSE ("EndCurrentLine")] -> w757
                    frame False {
                      n815 = local read "EndCurrentLine"() -> (w762:bool)
                      n816 = case shown="True" w762 {
                        frame False {
                        }
                        frame True {
                          n817 = local write "OnlyStopLineONCE Z"(TRUE ("EndCurrentLine")) -> ()
                        }
                      }
                    }
                    frame True {
                    }
                  }
                  n818 = local read "External Stop"() -> (w760:bool)
                  n819 = Or(x=w755, y=w757) -> (x .or. y?=w759:bool)
                  n820 = Or(x=w760, y=w759) -> (x .or. y?=w756:bool)
                }
              }
              n821 = local write "StopMoveZ"(w358) -> ()
            }
          }
          frame True {
          }
        }
        n822 = case shown="False" w215 {
          tunnel: w213 -> [w292 _]
          frame False {
            n823 = while {
              shift-right: [w294] -> _
              shift-left: w292 -> [w297]
              stop <- w293 stop-if-true
              n824 = flat-sequence {
                tunnel: w297 -> [w299]
                tunnel: [w300] -> w298
                tunnel: w298 -> [w325]
                tunnel: [w325] -> w296
                tunnel: [w321] -> w295
                tunnel: [w350] -> w294
                tunnel: w296 -> [w350]
                tunnel: w295 -> [w344]
                tunnel: [w345] -> w293
                frame #0 {
                  n825 = local read "Internal Pause"() -> (w302:bool)
                  n826 = local read "External Pause"() -> (w303:bool)
                  n827 = Or(x=w303, y=w302) -> (x .or. y?=w301:bool)
                  n828 = case shown="True" w301 {
                    tunnel: w299 -> [w304 w307]
                    tunnel: [w304 w305] -> w300
                    frame False {
                    }
                    frame True {
                      n829 = global read "Tick Count.vi" "Tick Count"() -> (w306:u64)
                      n830 = while {
                        shift-right: [w319] -> w305
                        shift-left: w307 -> [w311]
                        shift-right: [w314] -> _
                        shift-left: w306 -> [w313]
                        stop <- w308 stop-if-true
                        n831 = local read "External Pause"() -> (w318:bool)
                        n832 = local read "Internal Pause"() -> (w316:bool)
                        n833 = global read "Tick Count.vi" "Tick Count"() -> (w314:u64)
                        n834 = local read "External Stop"() -> (w310:bool)
                        n835 = Not(x=w318) -> (.not. x?=w317:bool)
                        n836 = Not(x=w316) -> (.not. x?=w315:bool)
                        n837 = Subtract(x=w314, y=w313) -> (x-y=w312:u64)
                        n838 = And(x=w317, y=w315) -> (x .and. y?=w309:bool)
                        n839 = Add(x=w312, y=w311) -> (x+y=w319:u64)
                        n840 = Or(x=w309, y=w310) -> (x .or. y?=w308:bool)
                      }
                    }
                  }
                }
                frame #1 {
                  n841 = global read "Tick Count.vi" "Tick Count"() -> (w324:u64)
                  n842 = Subtract(x=w324, y=w325) -> (x-y=w322:u64)
                  n843 = To Fixed-Point(number=w322) -> (fixed-point=w323:fxp<+,64,64>)  [unwired: 1 in]
                  n844 = case shown="True" "Change V on Fly 2" {
                    tunnel: w323 -> [w330 _]
                    tunnel: [w329 FALSE ("Finished Move")] -> w321
                    frame False {
                      n845 = local read "V2 END"() -> (w327:i16)
                      n846 = local read "Jump V2"() -> (w328:bool)
                      n847 = case shown="True" w328 {
                        tunnel: w327 -> [w339 w340]
                        tunnel: [w338 w340] -> w326
                        tunnel: w330 -> [w337 _]
                        tunnel: [w336 TRUE ("Finished Move")] -> w329
                        frame False {
                          n848 = local read "ExpandVelScaller V2"() -> (w331:i16)
                          n849 = local read "V2 VEl"() -> (w334:i16)
                          n850 = local read "V2 START"() -> (w335:i16)
                          n851 = Number To Boolean Array(number=w334) -> (Boolean array=w333:bool[])
                          n852 = Boolean Array To Number(Boolean array=w333) -> (number=w332:fxp<+/-,16,16>)
                          n853 = call "LinearMove.vi"("Time"=w337, "Start"=w335, "End"=w339, "Velocity"=w332, "ExpandVelScaller"=w331) -> ("OutPosition"=w338:i16, "Finished Move"=w336:bool)  [unwired: 13 in]
                        }
                        frame True {
                        }
                      }
                      n854 = local write "Applied Voltage 2"(w326) -> ()
                      n855 = xnode "FPGA I/O Node"("Connector0/AO4"=w326) -> ()  [unwired: 1 in, 1 out]
                    }
                    frame True {
                      n856 = local write "Applied Voltage 2"("V2 on Fly") -> ()
                      n857 = xnode "FPGA I/O Node"("Connector0/AO4"="V2 on Fly") -> ()  [unwired: 1 in, 1 out]
                    }
                  }
                }
                frame #2 {
                  n858 = local read "OnlyStopLineONCE V2"() -> (w346:bool)
                  n859 = case shown="False" w346 {
                    tunnel: [w351 FALSE ("EndCurrentLine")] -> w347
                    frame False {
                      n860 = local read "EndCurrentLine"() -> (w351:bool)
                      n861 = case shown="True" w351 {
                        frame False {
                        }
                        frame True {
                          n862 = local write "OnlyStopLineONCE V2"(TRUE ("EndCurrentLine")) -> ()
                        }
                      }
                    }
                    frame True {
                    }
                  }
                  n863 = Or(x=w344, y=w347) -> (x .or. y?=w349:bool)
                  n864 = local read "External Stop"() -> (w348:bool)
                  n865 = Or(x=w348, y=w349) -> (x .or. y?=w345:bool)
                }
              }
              n866 = local write "StopMoveV2"(w293) -> ()
            }
          }
          frame True {
          }
        }
      }
    }
  }
  n867 = node-c288(w2) -> ()
